vi "UHR-Fleezers Control (fpga) - 11.1.vi"() -> ()   [LabVIEW 2012]
doc: "UHR-Fleezers Instrument Control Code (fpga)"
uses:
  <vilib>/Platform/TimedLoop/XDataNode/timing_clust.ctl
  <vilib>/Platform/TimedLoop/XDataNode/nitl_modes.ctl
  <vilib>/Platform/TimedLoop/XDataNode/wakeup.ctl
  <vilib>/rvi/eio/common/nirviEmuTemplateMethod_errors.vi
  <vilib>/rvi/interface/RandomDataEmulation/nirviRandomDataFPGAFIFO.vi
  <vilib>/rvi/interface/RandomDataEmulation/niFpgaRandomDataHandleErrors.vi
  <vilib>/rvi/Emulation/niFpgaSctlEmulationGetInTimedLoop.vi
  <vilib>/rvi/Emulation/niFpgaSctlEmulationGlobalWrite.vi
  <vilib>/rvi/Emulation/niFpgaSctlEmulationRegisterWithScheduler.vi
  <vilib>/rvi/Emulation/niFpgaSctlEmulationScheduler.vi
  <vilib>/Platform/TimedLoop/XDataNode/XDataNode.xnode
  <vilib>/eio/EIONode/EIONode.xnode
  <vilib>/eio/EIOMethodNode/EIOMethodNode.xnode
  <vilib>/rvi/DataTransferAndStorage/Container/XNode/niFpgaContainer.xnode
  <vilib>/rvi/interface/RandomDataEmulation/nirviRandomDataFpgaReadWriteTemplate.vi
  <vilib>/addons/control/pid/fpga.llb/XNode/niFpgaPID.xnode
  <vilib>/Platform/TimedLoop/XDataNode/XDNodeRunTimeDep.lvlib
panel:
  in  "Tab Control":T1(tab)=enum."Force FB"
  in  "Set 3":bool
  in  "Set 2":bool=TRUE
  in  "Set 1":bool=TRUE
  in  "Trap Pos to FIFO":bool
  in  "N of AI1 Int Acq Sets":i16=2 min=1 max=3 step=1
  out "AI Late Counter":u16
  in  "ai count":u32=400
  out "AI late?":bool
  in  "+ phase":bool
  in  "Phase count adjustment":i16
  out "Relative phase":i16
  in  "AI to FIFO":bool
  out "BD1 Frequency Out 1":u64
  out "BD1 Frequency Out 2":u64
  out "Trap Pos FIFO Timeout":u16
  out "Trap AI FIFO Timeout":u16
  in  "Trap FIFO Set Timeout":i32
  in  "Tab Control 2":T2(tab)
  in  "RD":bool
  in  "FB1 output high":i16=3000
  in  "FB1 output low":i16
  in  "D1":i16
  in  "I1":i16=5
  in  "P1":i16=10
  in  "Swap F1 and F2":bool
  in  "Cont. Scan":bool
  in  "Abort scan":bool
  in  "Cycles per step":u64
  in  "Scan BD":bool
  in  "Number of scans":u16
  in  "Scan steps":u64
  in  "Scan freq.  increment":i64
  out "Scanning":bool
  in  "Start scan":bool
  in  "OSK Bd 1":bool
  in  "Reset Bd 1":bool
  in  "PMODE":bool
  in  "Direct RF Box \nCommunication":bool
  in  "Data BD 2":u8 format="%08b"
  in  "Data BD 1":u8 format="%08b"
  in  "Address":u8 format="%02x"
  in  "Update Data":bool
  in  "FPGA Controls\n RF Box":bool
  in  "Number Interlace Cycles":u8=2 min=1 max=3
  in  "Interlace Off Parameters":u8=1 min=1 max=3
  in  "Interlace ON/OFF":bool
  out "DIO Relative phase":i16
  in  "Phase count adjustment (DIO)":i16
  in  "+ phase (DIO)":bool
  out "DIO Late Counter":u16
  out "DIO Late?":bool
  in  "DIO count 1 (ticks)":u32=400
  in  "DIO count 2 (ticks)":u32=400
  in  "DIO count 3 (ticks)":u32=400
  out "AI2 Y Sum Set 2":i16
  out "AI2 Y Sum Set 1":i16
  in  "FB Setpoint Set 1":i16 min=0 step=1
  in  "FB Reset Set 1":bool
  in  "FB On/Off Set 1":bool
  in  "FB Reset Set 2":bool
  in  "FB On/Off Set 2":bool
  in  "FB Setpoint Set 2":i16 min=0 step=1
  out "Scan I":u64
  in  "Amp switch delay":u16=5
  in  "BD 2 Amplitude 1":u16
  in  "BD 1 Amplitude 1":u16
  in  "BD 2 Frequency 1":u64
  in  "BD 1 Frequency 1":u64
  in  "BD 2 Amplitude 2":u16
  in  "BD 1 Amplitude 2":u16
  in  "BD 2 Frequency 2":u64
  in  "BD 1 Frequency 2":u64
  in  "BD 2 Amplitude 3":u16
  in  "BD 1 Amplitude 3":u16
  in  "BD 2 Frequency 3":u64
  in  "BD 1 Frequency 3":u64
  in  "FB2 output high":fxp<+/-,16,1>=0.999969482421875
  in  "FB2 output low":fxp<+/-,16,1>=-1.0
  in  "P2":fxp<+/-,16,8> format="%.11g"
  in  "I2":fxp<+/-,16,8>=10.0 format="%.11g"
  in  "D2":fxp<+/-,16,8> format="%.11g"
  in  "Negate Diff?":bool
  in  "Diff FB Measurement?":bool
  in  "FB Trig Integrate":u32=1
  out "TTrig?":bool
  in  "TTrig Negate Pos":bool=TRUE
  out "Trap Pos FB Int Signal":fxp<+/-,24,9> format="%.18g"
  out "Trap Pos FB Int-Norm Signal":fxp<+/-,16,1> format="%.16g"
  in  "FPGA TTrig Thresh":i64
  in  "FPGA Trap Trig":bool
  out "Trap Pos FB Action":i64
  in  "Trap Pos. FB Offset Factor":i64
  in  "Trap Pos. FB Mult Factor":i64=2
  in  "Trap Pos. FB Reset":bool
  in  "Trap Pos FB Monitor T1 or T2":bool
  in  "AI1 X Scale":u16
  in  "Trap Pos FB Int Count":u16=100
  in  "Trap Pos FB Negate Action":bool
  out "AI1 X Set 2":fxp<+/-,16,1>
  out "AI1 X Set 1":fxp<+/-,16,1>
  in  "Trap Pos. FB SP":fxp<+/-,16,1>
  in  "Force feedback":bool
  out "TTrig Sig":i64
  out "TTrig Fin Thresh":i64
  in  "1D or 2D Scan?":bool
  in  "Abort scan (MCL)":bool
  in  "MCL Scan Axis":bool
  in  "Cont. Scan (MCL)":bool
  out "Scan I (MCL)":u64
  in  "Number of scans (MCL)":u16
  out "Scanning MCL":bool
  in  "Scan steps (MCL)":u64
  in  "Cycles per step (MCL)":u64
  in  "Scan freq.  increment (MCL)":i16
  in  "Start scan (MCL)":bool
  in  "AO2":i16
  in  "AO1":i16
  out "MCL Late Counter":u16
  out "MCL Late?":bool
  in  "MCL count":u32=800
  out "MCL Relative Phase":i16
  in  "Phase count adjustment (MCL)":i16
  in  "+ phase (MCL)":bool
  in  "APD Gate Operating Mode":u8 max=2 step=1
  in  "Invert APD Gate":bool
  in  "APD Gate OFF Count":u32=100
  in  "APD Gate ON Count":u32=300
  out "APD 1 Gate Late Counter":u16
  out "APD 1 Gate Late?":bool
  out "APD 1 Gate Relative Phase":i16
  in  "Phase count adjustment (APD 1 Gate)":i16
  in  "+ phase (APD 1 Gate)":bool
  out "APD 2 Counts 0":u32
  out "APD 2 Counts 1":u32
  out "APD 1 Counts 0":u32
  out "APD 1 Counts 1":u32
  out "APD1 out state":bool
  in  "APD 2 AO scale factor":i16=1
  in  "APD 1 AO scale factor":i16=1
  in  "APD to FIFO":bool
  in  "APD Acq Rate Count":u32=20000000
  out "APD Acq Late Counter":u16
  out "APD Acq Late?":bool
  out "APD Acq Relative Phase":i16
  in  "Phase Count Adjustment (APD Acq)":i16
  in  "+ phase (APD Acq)":bool
  in  "Phase count adjustment (APD 2 Gate)":i16
  out "APD 2 Gate Late Counter":u16
  out "APD 2 Gate Late?":bool
  out "APD 2 Gate Relative Phase":i16
  in  "+ phase (APD 2 Gate)":bool
  out "APD2 out state":bool
  in  "D3":i16
  in  "I3":i16=5
  in  "P3":i16=10
  in  "Green Filter Flipper":bool
  in  "Green FB Count":u32=1200
  out "Green Late Counter":u16
  out "Green FB Late?":bool
  out "Green FB Relative Phase":i16
  in  "Phase count adjustment (Green FB)":i16=10
  in  "+ phase (Green FB)":bool
  out "Green FB Sum":i16
  in  "Green int current ON count adj":u32=150
  in  "Current Out":u16=30000
  in  "Green FB On/Off":bool
  in  "Green FB Setpoint":i16=250 min=0 step=1
  in  "Green FB Reset":bool
  in  "Operating Mode 2":u8=2 max=2 step=1
  in  "Invert GI 2":bool
  in  "Green interlace OFF count 2":u32=900
  in  "Green interlace ON count 2":u32=300
  out "GI Late Counter 2":u16
  out "GI Late? 2":bool
  out "GI Relative phase 2":i16
  in  "Phase count adjustment (GI) 2":i16=20
  in  "+ phase (GI) 2":bool
  in  "Green interlace OFF count":u32=100
  out "GI Relative phase":i16
  in  "Phase count adjustment (GI)":i16
  in  "+ phase (GI)":bool
  out "GI Late?":bool
  in  "Green interlace ON count":u32=300
  out "GI Late Counter":u16
  in  "Invert GI":bool
  in  "Operating Mode":u8 max=2 step=1
  in  "+ phase (RI)":bool
  out "RI Relative phase":i16
  out "RI Late?":bool
  out "RI Late Counter":u16
  in  "Red interlace ON count":u32=300
  in  "Red interlace OFF count":u32=100
  in  "Invert RI":bool
  in  "Red Laser Operating Mode":u8 max=2 step=1
  in  "Phase count adjustment (RI)":i16
  out "Red FB Intensity":i16
  in  "Phase count adjustment (Red FB)":i16=10
  in  "Red FB Count":u32=1200
  out "Red Late Counter":u16
  out "Red FB Late?":bool
  out "Red FB Relative Phase":i16
  in  "+ phase (Red FB)":bool
  out "Green FB Sum 2":i16
  in  "Phase count adjustment (GI) 3":i16=20
  in  "Green int current ON count adj 2":u32=150
  in  "Current Out 2":u16=30000
  in  "Green FB On/Off 2":bool
  in  "D3 2":i16
  in  "I3 2":i16=5
  in  "P3 2":i16=10
  in  "Green FB Setpoint 2":i16=250 min=0 step=1
  in  "Green FB Reset 2":bool
  in  "Operating Mode 3":u8=2 max=2 step=1
  in  "Invert GI 3":bool
  in  "Green interlace OFF count 3":u32=900
  in  "Green interlace ON count 3":u32=300
  out "GI Late Counter 3":u16
  out "GI Late? 3":bool
  out "GI Relative phase 3":i16
  in  "+ phase (GI) 3":bool
  # "Only one of these can be on\nat a time:"
  # "Raster Scan AOD"
  # "1 (X)"
  # "2 (Y)"
  # "IR Intensity Feedback (RF BD 1)"
  # "FB Gains Set 1"
  # "FB output range 1"
  # "FB Triggering Excitation Laser"
  # "Trap Pos. FB Gains"
  # "Trap Pos. FB Range"
  # "AO1 (Y)"
  # "2D"
  # "1D"
  # "AO2 (X)"
  # "APD AO for aligning"
  # "Detection Loop"
  # "Green fluorescent laser digital gate interlacing loop"
  # "0 Forced ON\n1 Forced OFF\n2 Interlacing"
  # "Green FB Gains"
  # "Red fluorescent laser digital gate interlacing loop"
  # "Detection Loop"
  # "0 Forced ON\n1 Forced OFF\n2 Interlacing"
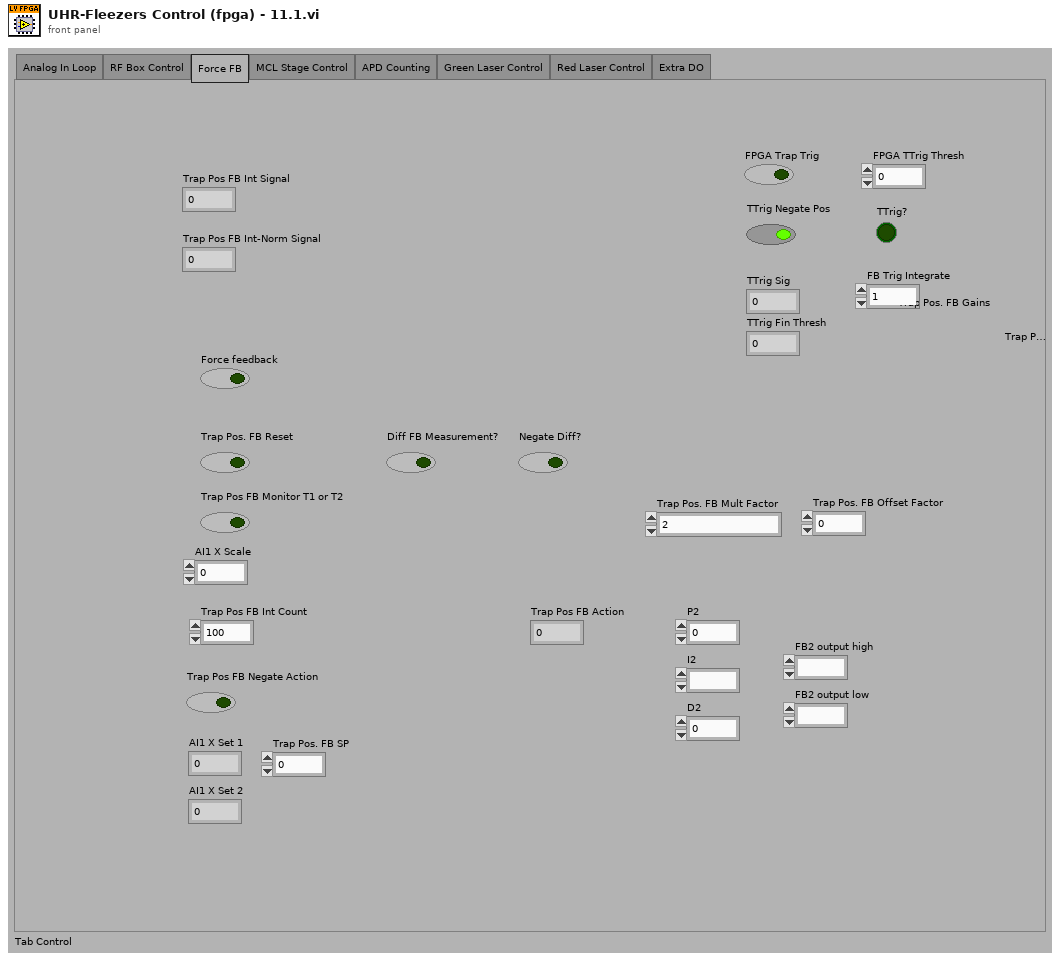
[diagram p1: front panel]
types:
  T1 = enum32{"Analog In Loop", "RF Box Control", "Force FB", "MCL Stage Control", "APD Counting", "Green Laser Control", "Red Laser Control", "Extra DO"}
  T2 = enum32{"Controls", "Interlacing Frequency and Amplitude Values"}
  T3 = typedef "XDNodeRunTimeDep.lvlib/timing_clust.ctl" = cluster{"Expected End [f-1]":u64, "Actual End [f-1]":u64, "Finished Late? [f-1]":bool, "Expected End [i-1]":u64, "Actual End [i-1]":u64, "Finished Late? [i-1]":bool, "Expected Start [i]":u64, "Actual Start [i]":u64, "Expected Start [f]":u64, "Actual Start [f]":u64, "Source Name":string, "Structure Name":string, "Period":i64, "Deadline":i64, "Offset":i64, "Start":i64, "Priority":i32, "Timeout":i32, "Mode":T4, "Wakeup Reason":T5, "Error":errorcluster, "Source Type":string, "Secondary Source Type":string, "Global End Time":u64, "Global Start Time":u64, "Frame Duration":u64, "Iteration Duration":u64, "Assigned CPU":i32, "I/O Scan Engine Mode":u32}
  T4 = typedef "XDNodeRunTimeDep.lvlib/nitl_modes.ctl" = enum32{"No Change", "Process missed periods, maintain original phase", "Discard missed periods, maintain original phase", "Process missed periods, ignore original phase", "Discard missed periods, ignore original phase"}
  T5 = typedef "XDNodeRunTimeDep.lvlib/wakeup.ctl" = enum32{"Normal", "Aborted", "Asynchronous wakeup", "Timing source error", "Timed loop error", "Timeout"}
  T6 = cluster{"proportional gain (Kc)":i16, "integral gain (Kc*Ts/Ti)":i16, "derivative gain (Kc*Td/Ts)":i16}
  T7 = cluster{"FB1 output high":i16, "FB1 output low":i16}
  T8 = cluster{"P2":fxp<+/-,16,8>, "I2":fxp<+/-,16,8>, "D2":fxp<+/-,16,8>}
  T9 = cluster{"FB2 output high":fxp<+/-,16,1>, "FB2 output low":fxp<+/-,16,1>}
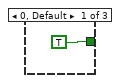
[diagram p3: hidden frame]
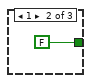
[diagram p4: hidden frame]
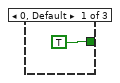
[diagram p5: hidden frame]
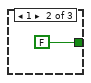
[diagram p6: hidden frame]
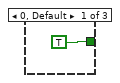
[diagram p7: hidden frame]
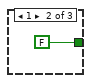
[diagram p8: hidden frame]
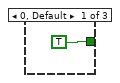
[diagram p10: hidden frame]
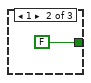
[diagram p11: hidden frame]
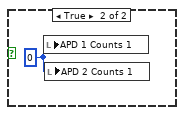
[diagram p12: hidden frame]
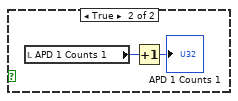
[diagram p14: hidden frame]
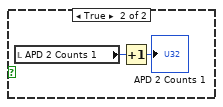
[diagram p15: hidden frame]
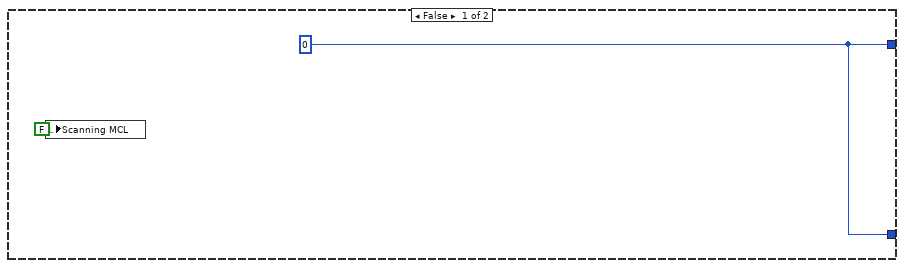
[diagram p16: hidden frame]
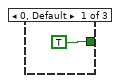
[diagram p17: hidden frame]
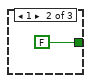
[diagram p18: hidden frame]
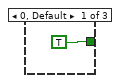
[diagram p19: hidden frame]
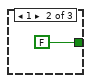
[diagram p20: hidden frame]
diagram:
  w3 = FALSE
  # "timing array current index"
  # "timing array"
  # "timing counter (phase adjusted here)"
  # "late counter"
  n1 = flat-sequence "FPGA initialization to do before running any of the loops" {
    tunnel: [u32 0 ("DIO count 3 (ticks)")] -> w1
    tunnel: [w10] -> _
    frame #0 {
      # "Start up expansion chassis early\nto avoid delays later"
      # "This pin controls udclk on the RF boards.\nWhen initially configuring the boards, this pin needs to be\nconfigured as a high impedance input.  Later it will be switched\nto an output."
      # "Initial setting of DIO data and \naddress to low (before reset).  \nThis needs to happen before the other\ncontrol method loops execute."
      n2 = xnode "FPGA I/O Node"("Chassis2/Mod4/AO0"=u16 0) -> ("Chassis2/Mod1/AI0"=w10:i16)  [unwired: 2 in, 2 out]
      n3 = xnode "FPGA I/O Method Node"("Enable"=FALSE) -> ()  [unwired: 1 in, 1 out]
      n4 = xnode "FPGA I/O Node"("Connector1/DIO0"=FALSE, "Connector1/DIO1"=FALSE, "Connector1/DIO2"=FALSE, "Connector1/DIO3"=FALSE, "Connector1/DIO4"=FALSE, "Connector1/DIO5"=FALSE, "Connector1/DIO6"=FALSE, "Connector1/DIO7"=FALSE, "Connector1/DIO8"=FALSE, "Connector1/DIO9"=FALSE, "Connector1/DIO10"=FALSE, "Connector1/DIO11"=FALSE, "Connector1/DIO12"=FALSE, "Connector1/DIO13"=FALSE, "Connector1/DIO15"=FALSE, "Connector1/DIO20"=FALSE, "Connector1/DIO21"=FALSE, "Connector1/DIO22"=FALSE, "Connector1/DIO23"=FALSE, "Connector1/DIO24"=FALSE, "Connector1/DIO25"=FALSE, "Connector1/DIO26"=FALSE, "Connector1/DIO27"=FALSE, "Connector1/DIO14"=FALSE) -> ()  [unwired: 24 in, 24 out]
    }
  }
  n5 = local read "AO1"() -> (w7:i16)
  n6 = local read "AO2"() -> (w6:i16)
  n7 = node-c288() -> (w5:T3)  [unwired: 1 in]
  n8 = timed-loop "RF box board DIO control: control bits" {
    timing: w5 -> [_]
    timing-out: [_] -> w4
    tunnel: [w40] -> _
    tunnel: w1 -> [w40]
    stop <- FALSE stop-if-true
    n9 = xnode "FPGA I/O Node"("Connector1/DIO16"="RD", "Connector1/DIO17"="PMODE", "Connector1/DIO18"="OSK Bd 1", "Connector1/DIO19"="Reset Bd 1", "Connector0/DIO3"="Green Filter Flipper") -> ()  [unwired: 5 in, 5 out]
  }
  n10 = while "RF box board DIO control: parallel communication" {
    shift-right: [w53] -> _
    shift-left: w1 -> [w52]
    shift-right: [w51] -> _
    shift-left: FALSE ("Swap F1 and F2") -> [w50]
    stop <- FALSE stop-if-true
    n11 = flat-sequence {
      tunnel: w50 -> [w57]
      tunnel: w52 -> [w55]
      tunnel: [w57] -> w49
      tunnel: [w56] -> w48
      tunnel: [w55] -> w47
      tunnel: [w63] -> w53
      tunnel: [w62] -> w51
      tunnel: w49 -> [w61]
      tunnel: w48 -> [w59]
      tunnel: w47 -> [w58]
      frame #0 {
        n12 = call "Loop Timer"("Count(Ticks)"=w55) -> ("Tick Count(Ticks)"=w56:u32)
      }
      frame #1 {
        n13 = flat-sequence {
          tunnel: ["FPGA Controls\n RF Box"] -> w60
          tunnel: w61 -> [w64]
          tunnel: [w104] -> w63
          tunnel: [w117] -> w62
          tunnel: w60 -> [w116]
          tunnel: w59 -> [w110]
          tunnel: w58 -> [w107]
          frame #0 {
            n14 = case shown="True" "FPGA Controls\n RF Box" {
              tunnel: w64 -> [_ w66]
              frame False {
              }
              frame True {
                n15 = flat-sequence {
                  tunnel: w66 -> [w72]
                  frame #0 {
                    n16 = First Call?() -> (First Call?: T/F=w67:bool)
                    n17 = case shown="True" w67 {
                      frame False {
                      }
                      frame True {
                        # "If first time data updated, be sure to set WR high and UDCLK low\nbefore setting data and address bits."
                        n18 = xnode "FPGA I/O Method Node"("Enable"=TRUE) -> ("FPGA I/O Out"=w69:refnum<k21>)  [unwired: 1 in]
                        n19 = xnode "FPGA I/O Node"("Connector1/DIO15"=TRUE) -> ()  [unwired: 1 in, 1 out]
                        n20 = xnode "FPGA I/O Node"("I/O Item"=FALSE ("Connector1/DIO30"), "FPGA I/O In"=w69) -> ()  [unwired: 1 out]
                      }
                    }
                  }
                  frame #1 {
                    n21 = flat-sequence {
                      tunnel: w72 -> [w73]
                      frame #0 {
                        # "switch frequency"
                        n22 = xnode "FPGA I/O Node"("Connector1/DIO36"=w73) -> ()  [unwired: 1 in, 1 out]
                      }
                      frame #1 {
                        n23 = call "Wait4"("Count(Ticks)"="Amp switch delay") -> ()  [unwired: 1 out]
                      }
                      frame #2 {
                        # "switch amplitude"
                        # "send udclk high"
                        n24 = xnode "FPGA I/O Node"("Connector1/DIO30"=TRUE ("Connector1/DIO15")) -> ()  [unwired: 1 in, 1 out]
                      }
                      frame #3 {
                        # "send udclk low"
                        n25 = xnode "FPGA I/O Node"("Connector1/DIO30"=FALSE ("Connector1/DIO15")) -> ()  [unwired: 1 in, 1 out]
                      }
                    }
                  }
                }
              }
            }
          }
          frame #1 {
            # "This is the prior cycle's on time"
            # "increment timing\nindex, reset to 0 if \nend of matrix"
            # "Reset to begginning (1) when number of cycles reached."
            # "timing index"
            # "build byte stacks for writing data\n(must correspond to addresses array constant)"
            # "Timing housekeeping"
            # "Adjust phase if late\n(maintains constant phase relationship between cycles)"
            n26 = Bundle("FB1 output high"="FB1 output high", "FB1 output low"="FB1 output low") -> (w77:T7)  [unwired: 1 in]
            n27 = Bundle("P1"="P1", "I1"="I1", "D1"="D1") -> (w78:cluster{"P1":i16, "I1":i16, "D1":i16})  [unwired: 1 in]
            n28 = feedback #1(u8 0 ("t")) -> (w113:u8)
            n29 = Increment(x=w113) -> (x+1=w157:u8)
            n30 = Increment(x="Number Interlace Cycles") -> (x+1=w152:u8)
            n31 = Equal?(x=w157, y=w152) -> (x = y?=w159:bool)
            n32 = Select(t=u8 1, s=w159, f=w157) -> (s? t:f=w112:u8)
            n33 = feedback-in #1(w112) -> ()
            n34 = Increment(x=w112) -> (x+1=w154:u8)
            n35 = Equal?(x=w154, y=w152) -> (x = y?=w155:bool)
            n36 = Select(t=u8 1, s=w155, f=w154) -> (s? t:f=w151:u8)
            n37 = Select(t=w151, s="Interlace ON/OFF", f="Interlace Off Parameters") -> (s? t:f=w135:u8)
            n38 = case shown="1, Default" w135 {
              tunnel: [w231 "BD 1 Frequency 2" "BD 1 Frequency 3"] -> w147
              tunnel: [w230 "BD 2 Frequency 2" "BD 2 Frequency 3"] -> w136
              tunnel: ["BD 2 Amplitude 1" "BD 2 Amplitude 2" "BD 2 Amplitude 3"] -> w92
              tunnel: [w219 w390 "BD 1 Amplitude 3"] -> w95
              tunnel: w78 -> [w193 w387 _]
              tunnel: w77 -> [w194 w386 _]
              frame 1, Default {
                w210 = fxp<+/-,24,9> 0.0 ("AI1 X Set 2")
                w203 = u16 0
                w226 = u64 0 ("f")
                # "This signal integration happens no matter what\nso that correct setpoints can be chosen before \nturning on the FB."
                # "Trap 1"
                n39 = local read "AI1 X Set 2"() -> (w206:fxp<+/-,16,1>)
                n40 = local read "AI1 X Set 1"() -> (w207:fxp<+/-,16,1>)
                n41 = local read "Scanning"() -> (w232:bool)
                n42 = Or(x=w232, y="Start scan") -> (x .or. y?=w224:bool)
                n43 = case shown="False" "Diff FB Measurement?" {
                  tunnel: w206 -> [w240 w249]
                  tunnel: w207 -> [w239 w250]
                  tunnel: [w237 w241] -> w208
                  frame False {
                    n44 = Select(t=w239, s="Trap Pos FB Monitor T1 or T2", f=w240) -> (s? t:f=w237:fxp<+/-,16,1>)
                  }
                  frame True {
                    n45 = Subtract(x=w250, y=w249) -> (x-y=w242:fxp<+/-,17,2>)
                    n46 = Not(x="Negate Diff?") -> (.not. x?=w248:bool)
                    n47 = Boolean To (0,1)(Boolean="Negate Diff?") -> (0, 1=w246:i16)
                    n48 = Boolean To (0,1)(Boolean=w248) -> (0, 1=w247:i16)
                    n49 = Negate(x=w246) -> (-x=w245:i16)
                    n50 = Add(x=w245, y=w247) -> (x+y=w243:i16)
                    n51 = Multiply(x=w243, y=w242) -> (x*y=w241:fxp<+/-,32,17>)
                  }
                }
                n52 = Not(x="Abort scan") -> (.not. x?=w222:bool)
                n53 = And(x=w222, y=w224) -> (x .and. y?=w221:bool)
                n54 = case "For raster scanning" shown="True" w221 {
                  tunnel: [u64 0 w376] -> w227
                  tunnel: "Start scan" -> [_ w361]
                  frame False {
                    n55 = local write "Scanning"(FALSE ("scanning")) -> ()
                  }
                  frame True {
                    w345 = i64 0
                    w344 = u64 0
                    # "scan incr."
                    # "freq. incr. mult."
                    # "count steps"
                    # "count number of cycles"
                    n56 = feedback #2(w344) -> (w373:u64)
                    n57 = Select(t=w344, s=w361, f=w373) -> (s? t:f=w375:u64)
                    n58 = Increment(x=w375) -> (x+1=w372:u64)
                    n59 = Greater?(x="Cycles per step", y=w372) -> (0:w354:bool)
                    n60 = Select(t=w372, s=w354, f=w344) -> (s? t:f=w371:u64)
                    n61 = feedback-in #2(w371) -> ()
                    n62 = feedback #3(w344) -> (w370:u64)
                    n63 = Select(t=w344, s=w361, f=w370) -> (s? t:f=w365:u64)
                    n64 = Increment(x=w365) -> (x+1=w369:u64)
                    n65 = Add(x="Scan steps", y="Scan steps") -> (x+y=w368:u64)
                    n66 = Select(t=w365, s=w354, f=w369) -> (s? t:f=w349:u64)
                    n67 = Greater?(x=w368, y=w349) -> (0:w348:bool)
                    n68 = Select(t=w349, s=w348, f=w344) -> (s? t:f=w366:u64)
                    n69 = feedback-in #3(w366) -> ()
                    n70 = Equal?(x="Scan steps", y=w349) -> (x = y?=w353:bool)
                    n71 = Greater?(x="Scan steps", y=w365) -> (0:w364:bool)
                    n72 = feedback #4(w345) -> (w367:i64)
                    n73 = Select(t=w345, s=w361, f=w367) -> (s? t:f=w351:i64)
                    n74 = Increment(x=w351) -> (x+1=w363:i64)
                    n75 = Decrement(x=w351) -> (x-1=w362:i64)
                    n76 = Select(t=w363, s=w364, f=w362) -> (s? t:f=w352:i64)
                    n77 = Select(t=w351, s=w353, f=w352) -> (s? t:f=w350:i64)
                    n78 = Select(t=w351, s=w354, f=w350) -> (s? t:f=w346:i64)
                    n79 = Select(t=w346, s=w348, f=w345) -> (s? t:f=w347:i64)
                    n80 = feedback-in #4(w347) -> ()
                    n81 = feedback #5(w344) -> (w360:u64)
                    n82 = Select(t=w344, s=w361, f=w360) -> (s? t:f=w356:u64)
                    n83 = Increment(x=w356) -> (x+1=w357:u64)
                    n84 = Select(t=w356, s=w348, f=w357) -> (s? t:f=w355:u64)
                    n85 = Greater?(x="Number of scans", y=w355) -> (0:w341:bool)
                    n86 = Multiply(x="Scan freq.  increment", y=w351) -> (x*y=w376:i64)
                    n87 = Select(t=TRUE, s="Cont. Scan", f=w341) -> (s? t:f=w340:bool)
                    "Scanning" <- w340
                    n88 = Select(t=w355, s=w340, f=w344) -> (s? t:f=w358:u64)
                    n89 = feedback-in #5(w358) -> ()
                    n90 = Increment(x=w355) -> (x+1=→"Scan I":u64)
                  }
                }
                n91 = feedback #6(w203) -> (w202:u16)
                n92 = Increment(x=w202) -> (x+1=w204:u16)
                n93 = Greater Or Equal?(x=w204, y="Trap Pos FB Int Count") -> (x >= y?=w195:bool)
                n94 = Select(t=w203, s=w195, f=w204) -> (s? t:f=w205:u16)
                n95 = feedback-in #6(w205) -> ()
                n96 = feedback #7(w210) -> (w209:fxp<+/-,24,9>)
                n97 = Add(x=w208, y=w209) -> (x+y=w201:fxp<+/-,24,9>)
                n98 = case "For intensity feedback" shown="True" "FB On/Off Set 1" {
                  tunnel: "BD 1 Amplitude 1" -> [w378 _]
                  tunnel: [w378 w382] -> w219
                  tunnel: w194 -> [_ w379]
                  tunnel: w193 -> [_ w380]
                  frame False {
                  }
                  frame True {
                    n99 = local read "AI2 Y Sum Set 1"() -> (w383:i16)
                    n100 = call "Slower PID.vi"("process variable"=w383, "reset?"="FB Reset Set 1", "setpoint"="FB Setpoint Set 1", "PID gains (x 2^8)"=w380, "output range"=w379) -> ("output"=w384:i16)  [unwired: 10 out]
                    n101 = To Unsigned Word Integer(number=w384) -> (unsigned 16bit integer=w382:u16)
                  }
                }
                n102 = Select(t=w210, s=w195, f=w201) -> (s? t:f=w213:fxp<+/-,24,9>)
                n103 = feedback-in #7(w213) -> ()
                n104 = Divide(x=w201, y="Trap Pos FB Int Count") -> (x/y=w196:fxp<+/-,16,1>)
                n105 = feedback #8(fxp<+/-,24,9> 0.0 ("AI1 X Set 2")) -> (w214:fxp<+/-,24,9>)
                n106 = Select(t=w201, s=w195, f=w214) -> (s? t:f=w215:fxp<+/-,24,9>)
                "Trap Pos FB Int Signal" <- w215
                n107 = feedback-in #8(w215) -> ()
                n108 = feedback #9(fxp<+/-,16,1> 0.0 ("Trap Pos FB Int-Norm Signal")) -> (w198:fxp<+/-,16,1>)
                n109 = Select(t=w196, s=w195, f=w198) -> (s? t:f=w197:fxp<+/-,16,1>)
                "Trap Pos FB Int-Norm Signal" <- w197
                n110 = feedback-in #9(w197) -> ()
                n111 = case "For position feedback" shown="True" "Force feedback" {
                  tunnel: [i64 0 w256] -> w216
                  tunnel: w196 -> [_ w253]
                  tunnel: w195 -> [_ w252]
                  frame False {
                  }
                  frame True {
                    n112 = feedback #10(i64 0) -> (w255:i64)
                    n113 = case shown="True" w252 {
                      tunnel: [w257 w271] -> w256
                      tunnel: w255 -> [w257 _]
                      tunnel: w253 -> [_ w265]
                      frame False {
                      }
                      frame True {
                        w275 = u32 0
                        n114 = Bundle("P2"="P2", "I2"="I2", "D2"="D2") -> (w261:T8)  [unwired: 1 in]
                        n115 = Bundle("FB2 output high"="FB2 output high", "FB2 output low"="FB2 output low") -> (w258:T9)  [unwired: 1 in]
                        n116 = xnode ("PID")("process variable"=w265, "reset?"="Trap Pos. FB Reset", "setpoint"="Trap Pos. FB SP", "PID gains"=w261, "output range"=w258) -> ("output"=w287:fxp<+/-,16,1>)
                        n117 = Negate(x=w287) -> (-x=w286:fxp<+/-,17,2>)
                        n118 = Select(t=w286, s="Trap Pos FB Negate Action", f=w287) -> (s? t:f=w283:fxp<+/-,17,2>)
                        n119 = Scale By Power Of 2(n=u32 15, x=u32 1) -> (x*2^n=w280:u32)
                        n120 = Multiply(x=w283, y=w280) -> (x*y=w279:fxp<+/-,17,17>)
                        n121 = To Quad Integer(1:w279) -> (0:w291:i64)
                        "Trap Pos FB Action" <- w291
                        n122 = Multiply(x=w291, y="Trap Pos. FB Mult Factor") -> (x*y=w289:i64)
                        n123 = Add(x=w289, y="Trap Pos. FB Offset Factor") -> (x+y=w271:i64)
                        n124 = feedback #11() -> (w272:i64)  [unwired: 1 in]
                        n125 = Add(x=w271, y=w272) -> (x+y=w269:i64)
                        n126 = feedback #12(w275) -> (w277:u32)
                        n127 = Increment(x=w277) -> (x+1=w266:u32)
                        n128 = Greater Or Equal?(x=w266, y="FB Trig Integrate") -> (x >= y?=w267:bool)
                        n129 = Select(t=i64 0, s=w267, f=w269) -> (s? t:f=w273:i64)
                        n130 = feedback-in #11(w273) -> ()
                        n131 = Select(t=w275, s=w267, f=w266) -> (s? t:f=w276:u32)
                        n132 = feedback-in #12(w276) -> ()
                        n133 = And(x=w267, y="FPGA Trap Trig") -> (x .and. y?=w274:bool)
                        n134 = case "Trap FB trigger excitation laser ON" shown="True" w274 {
                          tunnel: w269 -> [_ w295]
                          tunnel: w266 -> [_ w293]
                          frame False {
                          }
                          frame True {
                            n135 = Not(x="TTrig Negate Pos") -> (.not. x?=w302:bool)
                            n136 = Boolean To (0,1)(Boolean="TTrig Negate Pos") -> (0, 1=w300:i16)
                            n137 = Boolean To (0,1)(Boolean=w302) -> (0, 1=w301:i16)
                            n138 = Negate(x=w300) -> (-x=w299:i16)
                            n139 = Add(x=w299, y=w301) -> (x+y=w298:i16)
                            n140 = Multiply(x=w298, y=w295) -> (x*y=w297:i64)
                            "TTrig Sig" <- w297
                            n141 = Multiply(x="FPGA TTrig Thresh", y=w293) -> (x*y=w294:i64)
                            "TTrig Fin Thresh" <- w294
                            n142 = Greater Or Equal?(x=w297, y=w294) -> (x >= y?=w296:bool)
                            n143 = case shown="True" w296 {
                              frame False {
                              }
                              frame True {
                                w305 = TRUE ("Green FB On/Off")
                                w307 = u8 2 ("Operating Mode")
                                n144 = local write "Operating Mode 2"(w307) -> ()
                                n145 = local write "Operating Mode"(w307) -> ()
                                n146 = local write "Green FB On/Off"(w305) -> ()
                                n147 = local write "FPGA Trap Trig"(FALSE ("FPGA Trap Trig")) -> ()
                                "TTrig?" <- w305
                              }
                            }
                          }
                        }
                      }
                    }
                    n148 = feedback-in #10(w256) -> ()
                  }
                }
                n149 = Select(t=w226, s="Scan BD", f=w227) -> (s? t:f=w225:u64)
                n150 = Select(t=w227, s="Scan BD", f=w226) -> (s? t:f=w228:u64)
                n151 = Add(x=w225, y="BD 2 Frequency 1") -> (x+y=w230:u64)
                n152 = Compound Arithmetic op=ADD("BD 1 Frequency 1", w216, w228) -> (w231:u64)
                "BD1 Frequency Out 1" <- w231
              }
              frame 2 {
                # "Trap 2"
                n153 = case shown="True" "FB On/Off Set 2" {
                  tunnel: [w394 w397] -> w390
                  tunnel: "BD 1 Amplitude 2" -> [w394 _]
                  tunnel: w387 -> [_ w396]
                  tunnel: w386 -> [_ w395]
                  frame False {
                  }
                  frame True {
                    n154 = local read "AI2 Y Sum Set 2"() -> (w400:i16)
                    n155 = call "Slower PID.vi"("process variable"=w400, "reset?"="FB Reset Set 2", "setpoint"="FB Setpoint Set 2", "PID gains (x 2^8)"=w396, "output range"=w395) -> ("output"=w398:i16)  [unwired: 10 out]
                    n156 = To Unsigned Word Integer(number=w398) -> (unsigned 16bit integer=w397:u16)
                  }
                }
                "BD1 Frequency Out 2" <- "BD 1 Frequency 2"
              }
              frame 3 {
                # "Fluorescence period"
              }
            }
            n157 = feedback-in #13(w110) -> ()
            n158 = feedback #13(w110) -> (w109:u32)
            n159 = Select(t=w112, s="Interlace ON/OFF", f="Interlace Off Parameters") -> (s? t:f=w150:u8)
            n160 = Subtract(x=w110, y=w109) -> (x-y=w108:u32)
            n161 = Subtract "The error"(x=w108, y=w107) -> (x-y=w85:u32)
            n162 = case shown="1, Default" w150 {
              tunnel: ["DIO count 1 (ticks)" "DIO count 2 (ticks)" "DIO count 3 (ticks)"] -> w106
              frame 1, Default {
              }
              frame 2 {
              }
              frame 3 {
              }
            }
            n163 = Number To Boolean Array(number=w85) -> (Boolean array=w86:bool[])
            n164 = Or Array Elements(Boolean array=w86) -> (logical OR=w84:bool)
            "DIO Late?" <- w84
            n165 = Boolean To (0,1)(Boolean=w84) -> (0, 1=w91:i16)
            n166 = To Unsigned Word Integer(number=w91) -> (unsigned 16bit integer=w88:u16)
            n167 = feedback #14(u16 0) -> (w89:u16)
            n168 = Add(x=w88, y=w89) -> (x+y=w87:u16)
            "DIO Late Counter" <- w87
            n169 = feedback-in #14(w87) -> ()
            n170 = Subtract(x=w106, y=w85) -> (x-y=w105:u32)
            n171 = Split Number(x=w147) -> (hi(x)=w146:u32, lo(x)=w145:u32)
            n172 = Split Number(x=w136) -> (hi(x)=w141:u32, lo(x)=w140:u32)
            n173 = Boolean To (0,1)(Boolean="+ phase (DIO)") -> (0, 1=w102:i16)
            n174 = Split Number(x=w146) -> (lo(x)=w144:u16)  [unwired: 1 out]
            n175 = Split Number(x=w145) -> (hi(x)=w143:u16, lo(x)=w142:u16)
            n176 = Split Number(x=w141) -> (lo(x)=w139:u16)  [unwired: 1 out]
            n177 = Split Number(x=w140) -> (hi(x)=w138:u16, lo(x)=w137:u16)
            n178 = Split Number(x=w95) -> (hi(x)=w97:u8, lo(x)=w96:u8)
            n179 = Split Number(x=w92) -> (hi(x)=w94:u8, lo(x)=w93:u8)
            n180 = Split Number(x=w144) -> (hi(x)=w134:u8, lo(x)=w133:u8)
            n181 = Split Number(x=w143) -> (hi(x)=w132:u8, lo(x)=w131:u8)
            n182 = Split Number(x=w139) -> (hi(x)=w127:u8, lo(x)=w126:u8)
            n183 = Split Number(x=w142) -> (hi(x)=w130:u8, lo(x)=w129:u8)
            n184 = Split Number(x=w138) -> (hi(x)=w125:u8, lo(x)=w124:u8)
            n185 = Split Number(x=w137) -> (hi(x)=w123:u8, lo(x)=w122:u8)
            n186 = Multiply(x=w102, y="Phase count adjustment (DIO)") -> (x*y=w98:i16)
            n187 = feedback #15(i16 0) -> (w100:i16)
            n188 = Subtract(x=w100, y=w98) -> (x-y=w99:i16)
            "DIO Relative phase" <- w99
            n189 = feedback-in #15(w99) -> ()
            n190 = Add(x=w105, y=w98) -> (x+y=w104:u32)
            n191 = Build Array "BD 1 A Stack"(w97, w96) -> (w119:u8[])
            n192 = Build Array "BD 2 A Stack"(w94, w93) -> (w118:u8[])
            n193 = Build Array "BD 1 nu Stack"(w134, w133, w132, w131, w130, w129) -> (w128:u8[])
            n194 = Build Array "BD 2 nu Stack"(w127, w126, w125, w124, w123, w122) -> (w121:u8[])
            n195 = case shown="2" w135 {
              tunnel: [w185 w188] -> w117
              tunnel: [u8 10 u8 4] -> w120
              tunnel: "Swap F1 and F2" -> [w186 w188]
              frame 2 {
                # "F2"
                n196 = Not(x=w186) -> (.not. x?=w185:bool)
              }
              frame 1, Default {
                # "low chooses F1"
                # "F1"
              }
            }
            n197 = case "If FPGA is controlling (toggling) RF synth" shown="True" w116 {
              tunnel: w128 -> [_ w164]
              tunnel: w121 -> [_ w163]
              tunnel: w120 -> [_ w162]
              tunnel: w119 -> [_ w161]
              tunnel: w118 -> [_ w160]
              frame False {
              }
              frame True {
                # "Write next amp.\n(wait until beginning of next loop iteration to update)"
                n198 = flat-sequence "Update the next F1 and F2 frequency value (the actual frequency won't change until FSK is switched).\nThen load the next amplitude value into buffer, but don't update it until the next cycle." {
                  tunnel: w164 -> [w167]
                  tunnel: w163 -> [w166]
                  tunnel: w162 -> [w165]
                  tunnel: w161 -> [w178]
                  tunnel: w160 -> [w177]
                  frame #0 {
                    n199 = for {
                      tunnel: w167 -> [w173] mode=indexing
                      tunnel: w166 -> [w172] mode=indexing
                      tunnel: w165 -> [w170]
                      i -> [w171]
                      # "Write next freq."
                      n200 = To Unsigned Byte Integer(number=w171) -> (unsigned 8bit integer=w168:u8)
                      n201 = Add(x=w170, y=w168) -> (x+y=w169:u8)
                      n202 = call "write to RF synth bd.vi"("Address Byte"=w169, "BD 2 Byte"=w172, "BD 1 Byte"=w173) -> ()
                    }
                  }
                  frame #1 {
                    # "send udclk high"
                    n203 = xnode "FPGA I/O Node"("Connector1/DIO30"=TRUE ("Connector1/DIO15")) -> ()  [unwired: 1 in, 1 out]
                  }
                  frame #2 {
                    n204 = xnode "FPGA I/O Node"("Connector1/DIO30"=FALSE ("Connector1/DIO15")) -> ()  [unwired: 1 in, 1 out]
                  }
                  frame #3 {
                    n205 = for {
                      tunnel: w178 -> [w184] mode=indexing
                      tunnel: w177 -> [w183] mode=indexing
                      tunnel: u8 33 -> [w181]
                      i -> [w182]
                      n206 = To Unsigned Byte Integer(number=w182) -> (unsigned 8bit integer=w179:u8)
                      n207 = Add(x=w181, y=w179) -> (x+y=w180:u8)
                      n208 = call "write to RF synth bd.vi"("Address Byte"=w180, "BD 2 Byte"=w183, "BD 1 Byte"=w184) -> ()
                    }
                  }
                }
              }
            }
          }
        }
      }
    }
  }
  n209 = while "RF box board direct communication loop" {
    tunnel: w1 -> [_]
    stop <- FALSE stop-if-true
    n210 = case "Whether to use direct communication method (only use one method at a time)" shown="True" "Direct RF Box \nCommunication" {
      frame False {
      }
      frame True {
        n211 = case shown="True" "Update Data" {
          frame False {
          }
          frame True {
            n212 = flat-sequence {
              frame #0 {
                n213 = First Call?() -> (First Call?: T/F=w409:bool)
                n214 = case shown="True" w409 {
                  frame False {
                  }
                  frame True {
                    # "If first time data updated, be sure to set WR high\nbefore setting data and address bits."
                    n215 = flat-sequence {
                      frame #0 {
                        n216 = xnode "FPGA I/O Node"("Connector1/DIO15"=TRUE) -> ()  [unwired: 1 in, 1 out]
                      }
                      frame #1 {
                        n217 = call "Wait"("Count(Ticks)"=u8 40 ("DO Delay 3 (Ticks)")) -> ()  [unwired: 1 out]
                      }
                    }
                  }
                }
              }
              frame #1 {
                n218 = Number To Boolean Array(number="Address") -> (Boolean array=w458:bool[])
                n219 = Number To Boolean Array(number="Data BD 1") -> (Boolean array=w459:bool[])
                n220 = Number To Boolean Array(number="Data BD 2") -> (Boolean array=w428:bool[])
                n221 = Index Array(array=w459, index=7) -> (element=w443:bool)
                n222 = Index Array(array=w459, index=6) -> (element=w442:bool)
                n223 = Index Array(array=w459, index=5) -> (element=w441:bool)
                n224 = Index Array(array=w459, index=4) -> (element=w440:bool)
                n225 = Index Array(array=w459, index=3) -> (element=w439:bool)
                n226 = Index Array(array=w459, index=2) -> (element=w438:bool)
                n227 = Index Array(array=w459, index=1) -> (element=w437:bool)
                n228 = Index Array(array=w459, index=0) -> (element=w436:bool)
                n229 = Index Array(array=w458, index=5) -> (element=w435:bool)
                n230 = Index Array(array=w458, index=4) -> (element=w434:bool)
                n231 = Index Array(array=w458, index=3) -> (element=w433:bool)
                n232 = Index Array(array=w458, index=2) -> (element=w432:bool)
                n233 = Index Array(array=w458, index=1) -> (element=w431:bool)
                n234 = Index Array(array=w458, index=0) -> (element=w430:bool)
                n235 = Index Array(array=w428, index=7) -> (element=w419:bool)
                n236 = Index Array(array=w428, index=6) -> (element=w418:bool)
                n237 = Index Array(array=w428, index=5) -> (element=w417:bool)
                n238 = Index Array(array=w428, index=4) -> (element=w416:bool)
                n239 = Index Array(array=w428, index=3) -> (element=w415:bool)
                n240 = Index Array(array=w428, index=2) -> (element=w414:bool)
                n241 = Index Array(array=w428, index=1) -> (element=w413:bool)
                n242 = Index Array(array=w428, index=0) -> (element=w412:bool)
                n243 = xnode "FPGA I/O Node"("Connector1/DIO0"=w443, "Connector1/DIO1"=w442, "Connector1/DIO2"=w441, "Connector1/DIO3"=w440, "Connector1/DIO4"=w439, "Connector1/DIO5"=w438, "Connector1/DIO6"=w437, "Connector1/DIO7"=w436, "Connector1/DIO8"=w435, "Connector1/DIO9"=w434, "Connector1/DIO10"=w433, "Connector1/DIO11"=w432, "Connector1/DIO12"=w431, "Connector1/DIO13"=w430, "Connector1/DIO20"=w419, "Connector1/DIO21"=w418, "Connector1/DIO22"=w417, "Connector1/DIO23"=w416, "Connector1/DIO24"=w415, "Connector1/DIO25"=w414, "Connector1/DIO26"=w413, "Connector1/DIO27"=w412) -> ()  [unwired: 22 in, 22 out]
              }
              frame #2 {
                # "wait and then apply write signal"
                n244 = call "Wait2"("Count(Ticks)"=u8 40 ("DO Delay 1 (Ticks)")) -> ()  [unwired: 1 out]
              }
              frame #3 {
                # "sending bit low writes data to board buffer"
                n245 = xnode "FPGA I/O Node"("Connector1/DIO15"=FALSE) -> ()  [unwired: 1 in, 1 out]
              }
              frame #4 {
                # "wait then return write signal"
                n246 = call "Wait3"("Count(Ticks)"=u8 40 ("DO Delay 2 (Ticks)")) -> ()  [unwired: 1 out]
              }
              frame #5 {
                # "sending bit high makes ready to\nwrite more data"
                n247 = xnode "FPGA I/O Node"("Connector1/DIO15"=TRUE) -> ()  [unwired: 1 in, 1 out]
              }
            }
          }
        }
      }
    }
  }
  n248 = while "APD 1 Counter" {
    tunnel: w1 -> [_]
    stop <- FALSE stop-if-true
    n249 = flat-sequence {
      frame #0 {
        n250 = xnode "FPGA I/O Method Node"("FPGA I/O In"=refnum<k21> "Connector0/DIO0" ("APD 1 DO"), "Timeout"=-1) -> ()  [unwired: 2 out]
      }
      frame #1 {
        n251 = local read "APD1 out state"() -> (w469:bool)
        n252 = case shown="False" w469 {
          frame False {
            n253 = local read "APD 1 Counts 0"() -> (w471:u32)
            n254 = Increment(x=w471) -> (x+1=→"APD 1 Counts 0":u32)
          }
          frame True {
            n255 = local read "APD 1 Counts 1"() -> (w473:u32)
            n256 = Increment(x=w473) -> (x+1=→"APD 1 Counts 1":u32)
          }
        }
      }
    }
  }
  n257 = while "APD 2 Counter" {
    tunnel: w1 -> [_]
    stop <- FALSE stop-if-true
    n258 = flat-sequence {
      frame #0 {
        n259 = xnode "FPGA I/O Method Node"("FPGA I/O In"=refnum<k21> "Connector0/DIO1" ("APD 2 DO"), "Timeout"=-1) -> ()  [unwired: 2 out]
      }
      frame #1 {
        n260 = local read "APD2 out state"() -> (w477:bool)
        n261 = case shown="False" w477 {
          frame False {
            n262 = local read "APD 2 Counts 0"() -> (w479:u32)
            n263 = Increment(x=w479) -> (x+1=→"APD 2 Counts 0":u32)
          }
          frame True {
            n264 = local read "APD 2 Counts 1"() -> (w481:u32)
            n265 = Increment(x=w481) -> (x+1=→"APD 2 Counts 1":u32)
          }
        }
      }
    }
  }
  n266 = while "APD 2 Gating" {
    shift-right: [w485] -> _
    shift-left: w1 -> [w490]
    shift-right: [w484] -> _
    shift-left: w3 -> [w482]
    stop <- FALSE stop-if-true
    n267 = flat-sequence {
      tunnel: w490 -> [w493]
      tunnel: [w494] -> w488
      tunnel: [w493] -> w486
      tunnel: [w492] -> w483
      tunnel: w482 -> [w492]
      tunnel: [w497] -> w489
      tunnel: w488 -> [w497]
      tunnel: [w496] -> w487
      tunnel: w486 -> [w496]
      tunnel: w483 -> [w495]
      tunnel: [w515] -> w485
      tunnel: w489 -> [w526]
      tunnel: w487 -> [w524]
      tunnel: [w519] -> w484
      frame #0 {
        n268 = call "Loop Timer8"("Count(Ticks)"=w493) -> ("Tick Count(Ticks)"=w494:u32)
      }
      frame #1 {
        # "(need 4 channels/APD)"
        n269 = xnode "FPGA I/O Node"("Connector0/DIO8"=w495, "Connector0/DIO9"=w495, "Connector0/DIO10"=w495, "Connector0/DIO11"=w495) -> ()  [unwired: 4 in, 4 out]
      }
      frame #2 {
        n270 = local read "APD Gate ON Count"() -> (w508:u32)
        n271 = local read "APD Gate OFF Count"() -> (w507:u32)
        n272 = feedback #16(TRUE) -> (w521:bool)
        n273 = feedback-in #17(w526) -> ()
        n274 = feedback #17(w526) -> (w509:u32)
        n275 = Not(x=w521) -> (.not. x?=w518:bool)
        n276 = feedback-in #16(w518) -> ()
        n277 = Subtract(x=w526, y=w509) -> (x-y=w525:u32)
        n278 = Select(t=w508, s=w518, f=w507) -> (s? t:f=w523:u32)
        n279 = Subtract(x=w525, y=w524) -> (x-y=w500:u32)
        n280 = Subtract(x=w523, y=w500) -> (x-y=w514:u32)
        n281 = Number To Boolean Array(number=w500) -> (Boolean array=w499:bool[])
        n282 = Or Array Elements(Boolean array=w499) -> (logical OR=w498:bool)
        "APD 2 Gate Late?" <- w498
        n283 = Boolean To (0,1)(Boolean="+ phase (APD 2 Gate)") -> (0, 1=w512:i16)
        n284 = Multiply(x=w512, y="Phase count adjustment (APD 2 Gate)") -> (x*y=w510:i16)
        n285 = Boolean To (0,1)(Boolean=w498) -> (0, 1=w505:i16)
        n286 = Add(x=w514, y=w510) -> (x+y=w515:u32)
        n287 = To Unsigned Word Integer(number=w505) -> (unsigned 16bit integer=w502:u16)
        n288 = feedback #18(i16 0) -> (w517:i16)
        n289 = Subtract(x=w517, y=w510) -> (x-y=w516:i16)
        "APD 2 Gate Relative Phase" <- w516
        n290 = feedback-in #18(w516) -> ()
        n291 = feedback #19(u16 0) -> (w503:u16)
        n292 = Add(x=w502, y=w503) -> (x+y=w501:u16)
        "APD 2 Gate Late Counter" <- w501
        n293 = feedback-in #19(w501) -> ()
        n294 = local read "APD Gate Operating Mode"() -> (w506:u8)
        n295 = case shown="2" w506 {
          tunnel: [TRUE FALSE w532] -> w519
          tunnel: w521 -> [_ _ w530]
          frame 0, Default {
          }
          frame 1 {
          }
          frame 2 {
            n296 = local read "Invert APD Gate"() -> (w529:bool)
            n297 = Not(x=w530) -> (.not. x?=w531:bool)
            n298 = Select(t=w531, s=w529, f=w530) -> (s? t:f=w532:bool)
          }
        }
      }
    }
  }
  n299 = while "DAQ AI set 1" {
    shift-right: [w533] -> _
    shift-left: w1 -> [w538]
    stop <- FALSE stop-if-true
    n300 = flat-sequence {
      tunnel: w538 -> [w548]
      tunnel: [w549] -> w536
      tunnel: [w548] -> w535
      tunnel: [w559] -> w546
      tunnel: [w558] -> w545
      tunnel: [w557] -> w544
      tunnel: [w556] -> w543
      tunnel: [w555] -> w542
      tunnel: [w554] -> w541
      tunnel: [w553] -> w540
      tunnel: [w552] -> w539
      tunnel: [w551] -> w537
      tunnel: w536 -> [w551]
      tunnel: w535 -> [w550]
      tunnel: [w550] -> w534
      tunnel: [w588] -> w533
      tunnel: w546 -> [w615]
      tunnel: w545 -> [w580]
      tunnel: w544 -> [w581]
      tunnel: w543 -> [w614]
      tunnel: w542 -> [w604]
      tunnel: w541 -> [w603]
      tunnel: w540 -> [w602]
      tunnel: w539 -> [w601]
      tunnel: w537 -> [w598]
      tunnel: w534 -> [w595]
      frame #0 {
        n301 = call "Loop Timer3"("Count(Ticks)"=w548) -> ("Tick Count(Ticks)"=w549:u32)
      }
      frame #1 {
        n302 = xnode "FPGA I/O Node"("Connector1/DIO31"=TRUE ("Connector1/DIO33")) -> ("Connector0/AI0"=w559:i16, "Connector0/AI1"=w558:i16, "Connector0/AI2"=w557:i16, "Connector0/AI3"=w556:i16, "Connector0/AI4"=w555:i16, "Connector0/AI5"=w554:i16, "Connector0/AI6"=w553:i16, "Connector0/AI7"=w552:i16)  [unwired: 9 in, 9 out]
      }
      frame #2 {
        w584 = FALSE ("AI to FIFO")
        # "Adjust phase after data acquired if button pressed"
        n303 = feedback #20(i16 1) -> (w607:i16)
        n304 = Increment(x=w607) -> (x+1=w613:i16)
        n305 = Scale By Power Of 2(n="AI1 X Scale", x=w580) -> (x*2^n=w578:i16)
        n306 = Greater?(x=w613, y="N of AI1 Int Acq Sets") -> (0:w610:bool)
        n307 = Select(t=i16 1, s=w610, f=w613) -> (s? t:f=w612:i16)
        n308 = feedback-in #20(w612) -> ()
        n309 = Divide(x=w578, y=w581) -> (x/y=w577:fxp<+/-,16,1>)
        n310 = feedback #21(w584) -> (w582:bool)
        n311 = feedback #22(w584) -> (w600:bool)
        n312 = case shown="2" w607 {
          tunnel: w581 -> [w638 w645 _]
          tunnel: ["Set 1" "Set 2" "Set 3"] -> w605
          tunnel: ["AI to FIFO" w647 w652] -> w599
          tunnel: w600 -> [_ w647 w652]
          tunnel: ["Trap Pos to FIFO" w646 w651] -> w583
          tunnel: w582 -> [_ w646 w651]
          tunnel: w577 -> [w637 w644 _]
          tunnel: [w636 w642 FALSE] -> w564
          tunnel: [w635 w643 u64 0 ("BD1 Frequency Out 2")] -> w563
          frame 1, Default {
            n313 = local read "BD1 Frequency Out 1"() -> (w635:u64)
            n314 = Compound Arithmetic op=AND("Trap Pos to FIFO", "Set 1", "AI to FIFO") -> (w636:bool)
            "AI2 Y Sum Set 1" <- w638
            "AI1 X Set 1" <- w637
          }
          frame 2 {
            n315 = local read "BD1 Frequency Out 2"() -> (w643:u64)
            n316 = Compound Arithmetic op=AND(w646, "Set 2", w647) -> (w642:bool)
            "AI2 Y Sum Set 2" <- w645
            "AI1 X Set 2" <- w644
          }
          frame 3 {
          }
        }
        n317 = And(x=w605, y=w599) -> (x .and. y?=w606:bool)
        n318 = case shown="True" w606 {
          tunnel: w615 -> [_ w666]
          tunnel: w580 -> [_ w665]
          tunnel: w581 -> [_ w664]
          tunnel: w614 -> [_ w663]
          tunnel: w604 -> [_ w662]
          tunnel: w603 -> [_ w661]
          tunnel: w602 -> [_ w660]
          tunnel: w601 -> [_ w659]
          tunnel: 0 ("DMA buffer timeout") -> [_ w668]
          frame False {
          }
          frame True {
            n319 = Build Array(w666, w665, w664, w663, w662, w661, w660, w659) -> (w667:i16[])
            n320 = for {
              tunnel: w667 -> [w670] mode=indexing
              tunnel: w668 -> [w671]
              tunnel: [w669] -> w657 mode=indexing
              n321 = xnode ("FIFO Write")("Element"=w670, "Timeout"=w671) -> ("Timed Out?"=w669:bool)  [unwired: 1 in, 1 out]
            }
            n322 = Or Array Elements(Boolean array=w657) -> (logical OR=w654:bool)
            n323 = Boolean To (0,1)(Boolean=w654) -> (0, 1=w656:i16)
            n324 = feedback #23(u16 0) -> (w655:u16)
            n325 = Add(x=w656, y=w655) -> (x+y=w653:u16)
            "Trap AI FIFO Timeout" <- w653
            n326 = feedback-in #23(w653) -> ()
          }
        }
        n327 = feedback-in #21(w583) -> ()
        n328 = feedback-in #22(w599) -> ()
        n329 = case shown="True" w564 {
          tunnel: w563 -> [_ w621]
          tunnel: [u8 0 w618] -> w562
          frame False {
          }
          frame True {
            n330 = Split Number(x=w621) -> (hi(x)=w622:u32, lo(x)=w623:u32)
            n331 = Split Number(x=w622) -> (lo(x)=w624:u16)  [unwired: 1 out]
            n332 = Split Number(x=w623) -> (hi(x)=w625:u16, lo(x)=w626:u16)
            n333 = Build Array "BD 1 nu Stack"(w624, w625, w626) -> (w620:u16[])
            n334 = for {
              tunnel: w620 -> [w633] mode=indexing
              shift-right: [w629] -> w618
              shift-left: u8 0 -> [w630]
              n335 = xnode ("FIFO Method Node")("Element"=w633, "Timeout"="Trap FIFO Set Timeout") -> ("Timed Out?"=w632:bool)  [unwired: 1 in, 1 out]
              n336 = Boolean To (0,1)(Boolean=w632) -> (0, 1=w631:i16)
              n337 = To Unsigned Byte Integer(number=w631) -> (unsigned 8bit integer=w628:u8)
              n338 = Add(x=w628, y=w630) -> (x+y=w629:u8)
            }
          }
        }
        n339 = To Unsigned Word Integer(number=w562) -> (unsigned 16bit integer=w561:u16)
        n340 = feedback #24(u16 0) -> (w575:u16)
        n341 = Add(x=w561, y=w575) -> (x+y=w574:u16)
        "Trap Pos FIFO Timeout" <- w574
        n342 = feedback-in #24(w574) -> ()
        n343 = feedback-in #25(w598) -> ()
        n344 = feedback #25(w598) -> (w597:u32)
        n345 = Subtract(x=w598, y=w597) -> (x-y=w596:u32)
        n346 = xnode "FPGA I/O Node"("Connector1/DIO31"=FALSE ("Connector1/DIO34")) -> ()  [unwired: 1 in, 1 out]
        n347 = Subtract(x=w596, y=w595) -> (x-y=w566:u32)
        n348 = Boolean To (0,1)(Boolean="+ phase") -> (0, 1=w591:i16)
        n349 = Multiply(x=w591, y="Phase count adjustment") -> (x*y=w585:i16)
        n350 = Subtract(x="ai count", y=w566) -> (x-y=w589:u32)
        n351 = Number To Boolean Array(number=w566) -> (Boolean array=w567:bool[])
        n352 = feedback #26(i16 0) -> (w587:i16)
        n353 = Add(x=w589, y=w585) -> (x+y=w588:u32)
        n354 = Subtract(x=w587, y=w585) -> (x-y=w586:i16)
        "Relative phase" <- w586
        n355 = feedback-in #26(w586) -> ()
        n356 = Or Array Elements(Boolean array=w567) -> (logical OR=w565:bool)
        "AI late?" <- w565
        n357 = Boolean To (0,1)(Boolean=w565) -> (0, 1=w572:i16)
        n358 = To Unsigned Word Integer(number=w572) -> (unsigned 16bit integer=w569:u16)
        n359 = feedback #27(u16 0) -> (w570:u16)
        n360 = Add(x=w569, y=w570) -> (x+y=w568:u16)
        "AI Late Counter" <- w568
        n361 = feedback-in #27(w568) -> ()
      }
    }
  }
  n362 = while "MCL stage control" {
    shift-right: [w684] -> _
    shift-left: w1 -> [w687]
    shift-right: [w677] -> _
    shift-left: w7 -> [w674]
    shift-right: [w676] -> _
    shift-left: w6 -> [w672]
    stop <- FALSE stop-if-true
    n363 = flat-sequence {
      tunnel: w687 -> [w691]
      tunnel: [w692] -> w683
      tunnel: [w691] -> w681
      tunnel: [w690] -> w675
      tunnel: w674 -> [w690]
      tunnel: [w689] -> w673
      tunnel: w672 -> [w689]
      tunnel: w683 -> [w696]
      tunnel: [w696] -> w682
      tunnel: w681 -> [w695]
      tunnel: [w695] -> w680
      tunnel: w675 -> [w694]
      tunnel: w673 -> [w693]
      tunnel: w682 -> [w704]
      tunnel: w680 -> [w703]
      tunnel: [w704] -> w686
      tunnel: [w703] -> w685
      tunnel: [w702] -> w679
      tunnel: [w701] -> w678
      tunnel: [w776] -> w684
      tunnel: w686 -> [w783]
      tunnel: w685 -> [w780]
      tunnel: w679 -> [w778]
      tunnel: w678 -> [w777]
      tunnel: [w778] -> w677
      tunnel: [w777] -> w676
      frame #0 {
        n364 = call "Loop Timer5"("Count(Ticks)"=w691) -> ("Tick Count(Ticks)"=w692:u32)
      }
      frame #1 {
        n365 = xnode "FPGA I/O Node"("Connector0/AO1"=w694, "Connector0/AO2"=w693) -> ()  [unwired: 2 in, 2 out]
      }
      frame #2 {
        n366 = local read "Scanning MCL"() -> (w716:bool)
        n367 = Or(x=w716, y="Start scan (MCL)") -> (x .or. y?=w711:bool)
        n368 = Not(x="Abort scan (MCL)") -> (.not. x?=w709:bool)
        n369 = And(x=w709, y=w711) -> (x .and. y?=w708:bool)
        n370 = case "Raster scan" shown="True" w708 {
          tunnel: [w717 w760] -> w713
          tunnel: "Start scan (MCL)" -> [_ w745]
          tunnel: [w717 w721] -> w697
          frame False {
            w717 = i16 0
            n371 = local write "Scanning MCL"(FALSE ("scanning")) -> ()
          }
          frame True {
            w731 = i16 0
            w730 = u64 0
            # "scan incr."
            # "freq. incr. mult."
            # "count steps"
            # "count number of cycles"
            n372 = feedback #28(w730) -> (w757:u64)
            n373 = Select(t=w730, s=w745, f=w757) -> (s? t:f=w759:u64)
            n374 = Increment(x=w759) -> (x+1=w756:u64)
            n375 = Greater?(x="Cycles per step (MCL)", y=w756) -> (0:w740:bool)
            n376 = Select(t=w756, s=w740, f=w730) -> (s? t:f=w755:u64)
            n377 = feedback-in #28(w755) -> ()
            n378 = feedback #29(w730) -> (w754:u64)
            n379 = Select(t=w730, s=w745, f=w754) -> (s? t:f=w749:u64)
            n380 = Increment(x=w749) -> (x+1=w753:u64)
            n381 = Add(x="Scan steps (MCL)", y="Scan steps (MCL)") -> (x+y=w752:u64)
            n382 = Select(t=w749, s=w740, f=w753) -> (s? t:f=w735:u64)
            n383 = Greater?(x=w752, y=w735) -> (0:w734:bool)
            n384 = Select(t=w735, s=w734, f=w730) -> (s? t:f=w750:u64)
            n385 = feedback-in #29(w750) -> ()
            n386 = Equal?(x="Scan steps (MCL)", y=w735) -> (x = y?=w739:bool)
            n387 = Greater?(x="Scan steps (MCL)", y=w749) -> (0:w748:bool)
            n388 = feedback #30(w731) -> (w751:i16)
            n389 = Select(t=w731, s=w745, f=w751) -> (s? t:f=w737:i16)
            n390 = Increment(x=w737) -> (x+1=w747:i16)
            n391 = Decrement(x=w737) -> (x-1=w746:i16)
            n392 = Select(t=w747, s=w748, f=w746) -> (s? t:f=w738:i16)
            n393 = Select(t=w737, s=w739, f=w738) -> (s? t:f=w736:i16)
            n394 = Select(t=w737, s=w740, f=w736) -> (s? t:f=w732:i16)
            n395 = Select(t=w732, s=w734, f=w731) -> (s? t:f=w733:i16)
            n396 = feedback-in #30(w733) -> ()
            n397 = feedback #31(w730) -> (w744:u64)
            n398 = Select(t=w730, s=w745, f=w744) -> (s? t:f=w719:u64)
            n399 = Increment(x=w719) -> (x+1=w741:u64)
            n400 = Select(t=w719, s=w734, f=w741) -> (s? t:f=w720:u64)
            n401 = Greater?(x="Number of scans (MCL)", y=w720) -> (0:w727:bool)
            n402 = Multiply(x="Scan freq.  increment (MCL)", y=w737) -> (x*y=w760:i16)
            n403 = Select(t=TRUE, s="Cont. Scan (MCL)", f=w727) -> (s? t:f=w726:bool)
            "Scanning MCL" <- w726
            n404 = Select(t=w720, s=w726, f=w730) -> (s? t:f=w742:u64)
            n405 = feedback-in #31(w742) -> ()
            n406 = Increment(x=w720) -> (x+1=→"Scan I (MCL)":u64)
            n407 = To Word Integer(number=w719) -> (16bit integer=w722:i16)
            n408 = Multiply(x=w722, y="Scan freq.  increment (MCL)") -> (x*y=w721:i16)
          }
        }
        n409 = Select(t=w697, s="1D or 2D Scan?", f=i16 0) -> (s? t:f=w698:i16)
        n410 = Select(t=w698, s="MCL Scan Axis", f=w713) -> (s? t:f=w712:i16)
        n411 = Select(t=w713, s="MCL Scan Axis", f=w698) -> (s? t:f=w714:i16)
        n412 = Add(x=w712, y="AO2") -> (x+y=w701:i16)
        n413 = Add(x="AO1", y=w714) -> (x+y=w702:i16)
      }
      frame #3 {
        n414 = feedback-in #32(w783) -> ()
        n415 = feedback #32(w783) -> (w782:u32)
        n416 = Boolean To (0,1)(Boolean="+ phase (MCL)") -> (0, 1=w774:i16)
        n417 = Subtract(x=w783, y=w782) -> (x-y=w781:u32)
        n418 = Multiply(x=w774, y="Phase count adjustment (MCL)") -> (x*y=w770:i16)
        n419 = Subtract(x=w781, y=w780) -> (x-y=w762:u32)
        n420 = Subtract(x="MCL count", y=w762) -> (x-y=w772:u32)
        n421 = feedback #33(i16 0) -> (w771:i16)
        n422 = Subtract(x=w771, y=w770) -> (x-y=w769:i16)
        "MCL Relative Phase" <- w769
        n423 = feedback-in #33(w769) -> ()
        n424 = Number To Boolean Array(number=w762) -> (Boolean array=w763:bool[])
        n425 = Or Array Elements(Boolean array=w763) -> (logical OR=w761:bool)
        "MCL Late?" <- w761
        n426 = Boolean To (0,1)(Boolean=w761) -> (0, 1=w768:i16)
        n427 = Add(x=w772, y=w770) -> (x+y=w776:u32)
        n428 = To Unsigned Word Integer(number=w768) -> (unsigned 16bit integer=w765:u16)
        n429 = feedback #34(u16 0) -> (w766:u16)
        n430 = Add(x=w765, y=w766) -> (x+y=w764:u16)
        "MCL Late Counter" <- w764
        n431 = feedback-in #34(w764) -> ()
      }
    }
  }
  n432 = while "APD 1 Gating" {
    shift-right: [w788] -> _
    shift-left: w1 -> [w793]
    shift-right: [w787] -> _
    shift-left: w3 -> [w785]
    stop <- FALSE stop-if-true
    n433 = flat-sequence {
      tunnel: w793 -> [w796]
      tunnel: [w797] -> w791
      tunnel: [w796] -> w789
      tunnel: [w795] -> w786
      tunnel: w785 -> [w795]
      tunnel: [w800] -> w792
      tunnel: w791 -> [w800]
      tunnel: [w799] -> w790
      tunnel: w789 -> [w799]
      tunnel: w786 -> [w798]
      tunnel: [w814] -> w788
      tunnel: w792 -> [w829]
      tunnel: w790 -> [w826]
      tunnel: [w818] -> w787
      frame #0 {
        n434 = call "Loop Timer7"("Count(Ticks)"=w796) -> ("Tick Count(Ticks)"=w797:u32)
      }
      frame #1 {
        # "(need 4 channels/APD)"
        n435 = xnode "FPGA I/O Node"("Connector0/DIO4"=w798, "Connector0/DIO5"=w798, "Connector0/DIO6"=w798, "Connector0/DIO7"=w798) -> ()  [unwired: 4 in, 4 out]
      }
      frame #2 {
        n436 = feedback #35(TRUE) -> (w821:bool)
        n437 = feedback-in #36(w829) -> ()
        n438 = feedback #36(w829) -> (w828:u32)
        n439 = Not(x=w821) -> (.not. x?=w817:bool)
        n440 = feedback-in #35(w817) -> ()
        n441 = Subtract(x=w829, y=w828) -> (x-y=w827:u32)
        n442 = Select(t="APD Gate ON Count", s=w817, f="APD Gate OFF Count") -> (s? t:f=w823:u32)
        n443 = Subtract(x=w827, y=w826) -> (x-y=w802:u32)
        n444 = Subtract(x=w823, y=w802) -> (x-y=w813:u32)
        n445 = Number To Boolean Array(number=w802) -> (Boolean array=w803:bool[])
        n446 = Or Array Elements(Boolean array=w803) -> (logical OR=w801:bool)
        "APD 1 Gate Late?" <- w801
        n447 = Boolean To (0,1)(Boolean="+ phase (APD 1 Gate)") -> (0, 1=w811:i16)
        n448 = Boolean To (0,1)(Boolean=w801) -> (0, 1=w808:i16)
        n449 = Multiply(x=w811, y="Phase count adjustment (APD 1 Gate)") -> (x*y=w809:i16)
        n450 = To Unsigned Word Integer(number=w808) -> (unsigned 16bit integer=w805:u16)
        n451 = Add(x=w813, y=w809) -> (x+y=w814:u32)
        n452 = feedback #37(i16 0) -> (w816:i16)
        n453 = Subtract(x=w816, y=w809) -> (x-y=w815:i16)
        "APD 1 Gate Relative Phase" <- w815
        n454 = feedback-in #37(w815) -> ()
        n455 = feedback #38(u16 0) -> (w806:u16)
        n456 = Add(x=w805, y=w806) -> (x+y=w804:u16)
        "APD 1 Gate Late Counter" <- w804
        n457 = feedback-in #38(w804) -> ()
        n458 = case shown="2" "APD Gate Operating Mode" {
          tunnel: [TRUE FALSE w835] -> w818
          tunnel: w821 -> [_ _ w832]
          frame 0, Default {
          }
          frame 1 {
          }
          frame 2 {
            n459 = Not(x=w832) -> (.not. x?=w834:bool)
            n460 = Select(t=w834, s="Invert APD Gate", f=w832) -> (s? t:f=w835:bool)
          }
        }
      }
    }
  }
  n461 = while "Control APD data integration - stream to host" {
    shift-right: [w838] -> _
    shift-left: w1 -> [w843]
    stop <- FALSE stop-if-true
    n462 = flat-sequence {
      tunnel: w843 -> [w845]
      tunnel: [w846] -> w841
      tunnel: [w845] -> w839
      tunnel: [w854] -> w842
      tunnel: w841 -> [w854]
      tunnel: [w853] -> w840
      tunnel: w839 -> [w853]
      tunnel: [w852] -> w837
      tunnel: [w851] -> w836
      tunnel: [w888] -> w838
      tunnel: w842 -> [w900]
      tunnel: w840 -> [w897]
      tunnel: w837 -> [w881]
      tunnel: w836 -> [w880]
      frame #0 {
        n463 = call "Loop Timer6"("Count(Ticks)"=w845) -> ("Tick Count(Ticks)"=w846:u32)
      }
      frame #1 {
        n464 = flat-sequence {
          tunnel: [w856] -> w850
          tunnel: w850 -> [w858]
          tunnel: [w860] -> w849
          tunnel: [w859] -> w848
          tunnel: [w858] -> w847
          tunnel: [w866] -> w851
          tunnel: [w867] -> w852
          tunnel: w849 -> [w867]
          tunnel: w848 -> [w866]
          tunnel: w847 -> [w865]
          frame #0 {
            # "use two separate variable so each APD won't\nhave to wait to read"
            n465 = feedback #39(FALSE) -> (w855:bool)
            "APD1 out state" <- w855
            "APD2 out state" <- w855
            n466 = Not(x=w855) -> (.not. x?=w856:bool)
            n467 = feedback-in #39(w856) -> ()
          }
          frame #1 {
            n468 = local read "APD 1 Counts 1"() -> (w864:u32)
            n469 = local read "APD 1 Counts 0"() -> (w863:u32)
            n470 = local read "APD 2 Counts 1"() -> (w862:u32)
            n471 = local read "APD 2 Counts 0"() -> (w861:u32)
            n472 = Select(t=w864, s=w858, f=w863) -> (s? t:f=w860:u32)
            n473 = Select(t=w862, s=w858, f=w861) -> (s? t:f=w859:u32)
          }
          frame #2 {
            n474 = case shown="False" w865 {
              frame False {
                w868 = u32 0 ("APD 1 Counts 0")
                n475 = local write "APD 1 Counts 0"(w868) -> ()
                n476 = local write "APD 2 Counts 0"(w868) -> ()
              }
              frame True {
                w869 = u32 0 ("APD 1 Counts 1")
                n477 = local write "APD 1 Counts 1"(w869) -> ()
                n478 = local write "APD 2 Counts 1"(w869) -> ()
              }
            }
          }
        }
      }
      frame #2 {
        n479 = feedback-in #40(w900) -> ()
        n480 = feedback #40(w900) -> (w899:u32)
        n481 = Subtract(x=w900, y=w899) -> (x-y=w898:u32)
        n482 = Subtract(x=w898, y=w897) -> (x-y=w873:u32)
        n483 = case shown="True" "APD to FIFO" {
          tunnel: w881 -> [_ w903]
          tunnel: w880 -> [_ w901]
          frame False {
          }
          frame True {
            n484 = flat-sequence {
              tunnel: 0 ("Timeout") -> [w905]
              tunnel: w903 -> [w906]
              tunnel: [w905] -> w902
              tunnel: w902 -> [w908]
              tunnel: w901 -> [w907]
              frame #0 {
                n485 = xnode ("FIFO Write")("Element"=w906, "Timeout"=w905) -> ()  [unwired: 1 in, 2 out]
              }
              frame #1 {
                n486 = xnode ("FIFO Write")("Element"=w907, "Timeout"=w908) -> ()  [unwired: 1 in, 2 out]
              }
            }
          }
        }
        n487 = Subtract(x="APD Acq Rate Count", y=w873) -> (x-y=w889:u32)
        n488 = Number To Boolean Array(number=w873) -> (Boolean array=w874:bool[])
        n489 = Or Array Elements(Boolean array=w874) -> (logical OR=w872:bool)
        "APD Acq Late?" <- w872
        n490 = Boolean To (0,1)(Boolean=w872) -> (0, 1=w879:i16)
        n491 = To Unsigned Word Integer(number=w879) -> (unsigned 16bit integer=w876:u16)
        n492 = Boolean To (0,1)(Boolean="+ phase (APD Acq)") -> (0, 1=w885:i16)
        n493 = feedback #41(u16 0) -> (w877:u16)
        n494 = Add(x=w876, y=w877) -> (x+y=w875:u16)
        "APD Acq Late Counter" <- w875
        n495 = feedback-in #41(w875) -> ()
        n496 = Multiply(x=w885, y="Phase Count Adjustment (APD Acq)") -> (x*y=w882:i16)
        n497 = Add(x=w889, y=w882) -> (x+y=w888:u32)
        n498 = feedback #42(i16 0) -> (w887:i16)
        n499 = Subtract(x=w887, y=w882) -> (x-y=w884:i16)
        "APD Acq Relative Phase" <- w884
        n500 = feedback-in #42(w884) -> ()
        n501 = To Word Integer(number=w881) -> (16bit integer=w890:i16)
        n502 = To Word Integer(number=w880) -> (16bit integer=w891:i16)
        n503 = Multiply(x="APD 1 AO scale factor", y=w890) -> (x*y=w871:i16)
        n504 = Multiply(x="APD 2 AO scale factor", y=w891) -> (x*y=w870:i16)
        n505 = xnode "FPGA I/O Node"("Connector0/AO5"=w871, "Connector0/AO7"=w870) -> ()  [unwired: 2 in, 2 out]
      }
    }
  }
  n506 = while "532 nm green fluorescent laser interlacing (DO to IA 532 nm AOM ME amp)." {
    shift-right: [w912] -> _
    shift-left: w1 -> [w917]
    shift-right: [w911] -> _
    shift-left: FALSE -> [w909]
    stop <- FALSE stop-if-true
    n507 = flat-sequence {
      tunnel: w917 -> [w920]
      tunnel: [w921] -> w915
      tunnel: [w920] -> w913
      tunnel: [w919] -> w910
      tunnel: w909 -> [w919]
      tunnel: [w924] -> w916
      tunnel: w915 -> [w924]
      tunnel: [w923] -> w914
      tunnel: w913 -> [w923]
      tunnel: w910 -> [w922]
      tunnel: [w933] -> w912
      tunnel: w916 -> [w953]
      tunnel: w914 -> [w950]
      tunnel: [w942] -> w911
      frame #0 {
        n508 = call "Loop Timer4"("Count(Ticks)"=w920) -> ("Tick Count(Ticks)"=w921:u32)
      }
      frame #1 {
        n509 = xnode "FPGA I/O Node"("Connector1/DIO37"=w922, "Connector1/DIO38"=w922, "Connector1/DIO39"=w922) -> ()  [unwired: 3 in, 3 out]
      }
      frame #2 {
        n510 = feedback-in #43(w953) -> ()
        n511 = feedback #43(w953) -> (w952:u32)
        n512 = Subtract(x=w953, y=w952) -> (x-y=w951:u32)
        n513 = Subtract(x=w951, y=w950) -> (x-y=w926:u32)
        n514 = Number To Boolean Array(number=w926) -> (Boolean array=w927:bool[])
        n515 = Or Array Elements(Boolean array=w927) -> (logical OR=w925:bool)
        "GI Late?" <- w925
        n516 = Boolean To (0,1)(Boolean="+ phase (GI)") -> (0, 1=w938:i16)
        n517 = Multiply(x=w938, y="Phase count adjustment (GI)") -> (x*y=w935:i16)
        n518 = Boolean To (0,1)(Boolean=w925) -> (0, 1=w932:i16)
        n519 = To Unsigned Word Integer(number=w932) -> (unsigned 16bit integer=w929:u16)
        n520 = feedback #44(i16 0) -> (w936:i16)
        n521 = feedback #45(u16 0) -> (w930:u16)
        n522 = Add(x=w929, y=w930) -> (x+y=w928:u16)
        "GI Late Counter" <- w928
        n523 = feedback-in #45(w928) -> ()
        n524 = Subtract(x=w936, y=w935) -> (x-y=w934:i16)
        "GI Relative phase" <- w934
        n525 = feedback-in #44(w934) -> ()
        n526 = feedback #46(TRUE) -> (w945:bool)
        n527 = case shown="2" "Operating Mode" {
          tunnel: [TRUE FALSE w959] -> w942
          tunnel: w945 -> [_ _ w956]
          frame 0, Default {
          }
          frame 1 {
          }
          frame 2 {
            n528 = Not(x=w956) -> (.not. x?=w958:bool)
            n529 = Select(t=w958, s="Invert GI", f=w956) -> (s? t:f=w959:bool)
          }
        }
        n530 = Not(x=w945) -> (.not. x?=w941:bool)
        n531 = Select(t="Green interlace ON count", s=w941, f="Green interlace OFF count") -> (s? t:f=w947:u32)
        n532 = Subtract(x=w947, y=w926) -> (x-y=w939:u32)
        n533 = Add(x=w939, y=w935) -> (x+y=w933:u32)
        n534 = feedback-in #46(w941) -> ()
      }
    }
  }
  n535 = while "Green fluorescent laser interlacing (Current to IA 532 nm AOM ME amp)." {
    shift-right: [w965] -> _
    shift-left: w1 -> [w968]
    shift-right: [w962] -> _
    shift-left: u16 0 -> [w960]
    stop <- FALSE stop-if-true
    n536 = flat-sequence {
      tunnel: w968 -> [w971]
      tunnel: [w972] -> w967
      tunnel: [w971] -> w966
      tunnel: [w970] -> w961
      tunnel: w960 -> [w970]
      tunnel: [w975] -> w964
      tunnel: w967 -> [w975]
      tunnel: [w974] -> w963
      tunnel: w966 -> [w974]
      tunnel: w961 -> [w973]
      tunnel: [w984] -> w965
      tunnel: [w1001] -> w962
      tunnel: w964 -> [w1014]
      tunnel: w963 -> [w1011]
      frame #0 {
        n537 = call "Loop Timer10"("Count(Ticks)"=w971) -> ("Tick Count(Ticks)"=w972:u32)
      }
      frame #1 {
        n538 = xnode "FPGA I/O Node"("Chassis2/Mod4/AO0"=w973) -> ()  [unwired: 1 in, 1 out]
      }
      frame #2 {
        n539 = Subtract(x="Green interlace OFF count 2", y="Green int current ON count adj") -> (x-y=w993:u32)
        n540 = feedback-in #47(w1014) -> ()
        n541 = feedback #47(w1014) -> (w1013:u32)
        n542 = Add(x="Green int current ON count adj", y="Green interlace ON count 2") -> (x+y=w994:u32)
        n543 = Subtract(x=w1014, y=w1013) -> (x-y=w1012:u32)
        n544 = Subtract(x=w1012, y=w1011) -> (x-y=w977:u32)
        n545 = Number To Boolean Array(number=w977) -> (Boolean array=w978:bool[])
        n546 = Boolean To (0,1)(Boolean="+ phase (GI) 2") -> (0, 1=w990:i16)
        n547 = Or Array Elements(Boolean array=w978) -> (logical OR=w976:bool)
        "GI Late? 2" <- w976
        n548 = Boolean To (0,1)(Boolean=w976) -> (0, 1=w983:i16)
        n549 = Multiply(x=w990, y="Phase count adjustment (GI) 2") -> (x*y=w986:i16)
        n550 = To Unsigned Word Integer(number=w983) -> (unsigned 16bit integer=w979:u16)
        n551 = feedback #48(u16 0) -> (w981:u16)
        n552 = Add(x=w979, y=w981) -> (x+y=w980:u16)
        "GI Late Counter 2" <- w980
        n553 = feedback-in #48(w980) -> ()
        n554 = feedback #49(i16 0) -> (w987:i16)
        n555 = Subtract(x=w987, y=w986) -> (x-y=w985:i16)
        "GI Relative phase 2" <- w985
        n556 = feedback-in #49(w985) -> ()
        n557 = feedback #50(TRUE) -> (w1006:bool)
        n558 = case shown="2" "Operating Mode 2" {
          tunnel: [TRUE FALSE w1034] -> w995
          tunnel: w1006 -> [_ _ w1031]
          frame 0, Default {
          }
          frame 1 {
          }
          frame 2 {
            n559 = Not(x=w1031) -> (.not. x?=w1033:bool)
            n560 = Select(t=w1033, s="Invert GI 2", f=w1031) -> (s? t:f=w1034:bool)
          }
        }
        n561 = And(x=w995, y="Green FB On/Off") -> (x .and. y?=w996:bool)
        n562 = case shown="True" w996 {
          tunnel: "Current Out" -> [w1015 _]
          tunnel: [w1015 w1024] -> w1000
          frame False {
          }
          frame True {
            n563 = local read "Green FB Sum"() -> (w1020:i16)
            n564 = Bundle("P3"="P3", "I3"="I3", "D3"="D3") -> (w1016:cluster{"P3":i16, "I3":i16, "D3":i16})  [unwired: 1 in]
            n565 = call "Slower PID.vi"("process variable"=w1020, "reset?"="Green FB Reset", "setpoint"="Green FB Setpoint", "PID gains (x 2^8)"=w1016, "output range"=cluster{"output high":i16, "output low":i16} {"output high"=32767, "output low"=-32768} ("Green FB output range")) -> ("output"=w1027:i16)  [unwired: 10 out]
            n566 = To Long Integer(number=w1027) -> (32bit integer=w1021:i32)
            n567 = Add(x=w1021, y=32768) -> (x+y=w1023:i32)
            n568 = To Unsigned Word Integer(number=w1023) -> (unsigned 16bit integer=w1024:u16)
          }
        }
        n569 = Not(x=w1006) -> (.not. x?=w1003:bool)
        n570 = Select(t=w994, s=w1003, f=w993) -> (s? t:f=w1008:u32)
        n571 = Subtract(x=w1008, y=w977) -> (x-y=w988:u32)
        n572 = Add(x=w988, y=w986) -> (x+y=w984:u32)
        n573 = feedback-in #50(w1003) -> ()
        n574 = Boolean To (0,1)(Boolean=w995) -> (0, 1=w1002:i16)
        n575 = To Unsigned Word Integer(number=w1002) -> (unsigned 16bit integer=w999:u16)
        n576 = Multiply(x=w999, y=w1000) -> (x*y=w1001:u16)
      }
    }
  }
  n577 = while "532 nm green excitation laser intensity feedback measurement" {
    shift-right: [w1035] -> _
    shift-left: w1 -> [w1040]
    stop <- FALSE stop-if-true
    n578 = flat-sequence {
      tunnel: w1040 -> [w1042]
      tunnel: [w1043] -> w1038
      tunnel: [w1042] -> w1036
      tunnel: [w1047] -> w1039
      tunnel: w1038 -> [w1047]
      tunnel: [w1046] -> w1037
      tunnel: w1036 -> [w1046]
      tunnel: [w1059] -> w1035
      tunnel: w1039 -> [w1070]
      tunnel: w1037 -> [w1067]
      frame #0 {
        n579 = call "Loop Timer9"("Count(Ticks)"=w1042) -> ("Tick Count(Ticks)"=w1043:u32)
      }
      frame #1 {
        n580 = xnode "FPGA I/O Node"("Connector1/DIO35"=TRUE) -> ("Chassis2/Mod1/AI1"=→"Green FB Sum":i16)  [unwired: 2 in, 2 out]
      }
      frame #2 {
        n581 = feedback-in #51(w1070) -> ()
        n582 = feedback #51(w1070) -> (w1069:u32)
        n583 = Subtract(x=w1070, y=w1069) -> (x-y=w1068:u32)
        n584 = xnode "FPGA I/O Node"("Connector1/DIO35"=FALSE) -> ()  [unwired: 1 in, 1 out]
        n585 = Subtract(x=w1068, y=w1067) -> (x-y=w1049:u32)
        n586 = Subtract(x="Green FB Count", y=w1049) -> (x-y=w1063:u32)
        n587 = Number To Boolean Array(number=w1049) -> (Boolean array=w1050:bool[])
        n588 = Or Array Elements(Boolean array=w1050) -> (logical OR=w1048:bool)
        "Green FB Late?" <- w1048
        n589 = Boolean To (0,1)(Boolean="+ phase (Green FB)") -> (0, 1=w1061:i16)
        n590 = Boolean To (0,1)(Boolean=w1048) -> (0, 1=w1055:i16)
        n591 = Multiply(x=w1061, y="Phase count adjustment (Green FB)") -> (x*y=w1056:i16)
        n592 = Add(x=w1063, y=w1056) -> (x+y=w1059:u32)
        n593 = To Unsigned Word Integer(number=w1055) -> (unsigned 16bit integer=w1052:u16)
        n594 = feedback #52(i16 0) -> (w1058:i16)
        n595 = Subtract(x=w1058, y=w1056) -> (x-y=w1057:i16)
        "Green FB Relative Phase" <- w1057
        n596 = feedback-in #52(w1057) -> ()
        n597 = feedback #53(u16 0) -> (w1053:u16)
        n598 = Add(x=w1052, y=w1053) -> (x+y=w1051:u16)
        "Green Late Counter" <- w1051
        n599 = feedback-in #53(w1051) -> ()
      }
    }
  }
  n600 = node-c288(w4) -> ()
  n601 = while "Red fluorescent laser interlacing (Current to IA 532 nm AOM ME amp)." {
    shift-right: [w1076] -> _
    shift-left: _ -> [w1079]
    shift-right: [w1073] -> _
    shift-left: _ -> [w1071]
    stop <- FALSE stop-if-true
    n602 = flat-sequence {
      tunnel: w1079 -> [w1082]
      tunnel: [w1083] -> w1078
      tunnel: [w1082] -> w1077
      tunnel: [w1081] -> w1072
      tunnel: w1071 -> [w1081]
      tunnel: [w1086] -> w1075
      tunnel: w1078 -> [w1086]
      tunnel: [w1085] -> w1074
      tunnel: w1077 -> [w1085]
      tunnel: w1072 -> [w1084]
      tunnel: [w1095] -> w1076
      tunnel: [w1112] -> w1073
      tunnel: w1075 -> [w1125]
      tunnel: w1074 -> [w1122]
      frame #0 {
        n603 = call "Loop Timer2"("Count(Ticks)"=w1082) -> ("Tick Count(Ticks)"=w1083:u32)
      }
      frame #1 {
        n604 = xnode "FPGA I/O Node"("Chassis2/Mod4/AO0"=w1084) -> ()  [unwired: 1 in, 1 out]
      }
      frame #2 {
        n605 = Subtract(x="Green interlace OFF count 3", y="Green int current ON count adj 2") -> (x-y=w1104:u32)
        n606 = feedback-in #54(w1125) -> ()
        n607 = feedback #54(w1125) -> (w1124:u32)
        n608 = Add(x="Green int current ON count adj 2", y="Green interlace ON count 3") -> (x+y=w1105:u32)
        n609 = Subtract(x=w1125, y=w1124) -> (x-y=w1123:u32)
        n610 = Subtract(x=w1123, y=w1122) -> (x-y=w1088:u32)
        n611 = Number To Boolean Array(number=w1088) -> (Boolean array=w1089:bool[])
        n612 = Boolean To (0,1)(Boolean="+ phase (GI) 3") -> (0, 1=w1101:i16)
        n613 = Or Array Elements(Boolean array=w1089) -> (logical OR=w1087:bool)
        "GI Late? 3" <- w1087
        n614 = Boolean To (0,1)(Boolean=w1087) -> (0, 1=w1094:i16)
        n615 = Multiply(x=w1101, y="Phase count adjustment (GI) 3") -> (x*y=w1097:i16)
        n616 = To Unsigned Word Integer(number=w1094) -> (unsigned 16bit integer=w1090:u16)
        n617 = feedback #55(u16 0) -> (w1092:u16)
        n618 = Add(x=w1090, y=w1092) -> (x+y=w1091:u16)
        "GI Late Counter 3" <- w1091
        n619 = feedback-in #55(w1091) -> ()
        n620 = feedback #56(i16 0) -> (w1098:i16)
        n621 = Subtract(x=w1098, y=w1097) -> (x-y=w1096:i16)
        "GI Relative phase 3" <- w1096
        n622 = feedback-in #56(w1096) -> ()
        n623 = feedback #57(TRUE) -> (w1117:bool)
        n624 = case shown="2" "Operating Mode 3" {
          tunnel: [TRUE FALSE w1145] -> w1106
          tunnel: w1117 -> [_ _ w1142]
          frame 0, Default {
          }
          frame 1 {
          }
          frame 2 {
            n625 = Not(x=w1142) -> (.not. x?=w1144:bool)
            n626 = Select(t=w1144, s="Invert GI 3", f=w1142) -> (s? t:f=w1145:bool)
          }
        }
        n627 = And(x=w1106, y="Green FB On/Off 2") -> (x .and. y?=w1107:bool)
        n628 = case shown="True" w1107 {
          tunnel: "Current Out 2" -> [w1126 _]
          tunnel: [w1126 w1135] -> w1111
          frame False {
          }
          frame True {
            n629 = local read "Green FB Sum 2"() -> (w1131:i16)
            n630 = Bundle("P3 2"="P3 2", "I3 2"="I3 2", "D3 2"="D3 2") -> (w1127:cluster{"P3 2":i16, "I3 2":i16, "D3 2":i16})  [unwired: 1 in]
            n631 = call "Slower PID.vi"("process variable"=w1131, "reset?"="Green FB Reset 2", "setpoint"="Green FB Setpoint 2", "PID gains (x 2^8)"=w1127, "output range"=cluster{"output high":i16, "output low":i16} {"output high"=32767, "output low"=-32768} ("Green FB output range")) -> ("output"=w1138:i16)  [unwired: 10 out]
            n632 = To Long Integer(number=w1138) -> (32bit integer=w1132:i32)
            n633 = Add(x=w1132, y=32768) -> (x+y=w1134:i32)
            n634 = To Unsigned Word Integer(number=w1134) -> (unsigned 16bit integer=w1135:u16)
          }
        }
        n635 = Not(x=w1117) -> (.not. x?=w1114:bool)
        n636 = Select(t=w1105, s=w1114, f=w1104) -> (s? t:f=w1119:u32)
        n637 = Subtract(x=w1119, y=w1088) -> (x-y=w1099:u32)
        n638 = Add(x=w1099, y=w1097) -> (x+y=w1095:u32)
        n639 = feedback-in #57(w1114) -> ()
        n640 = Boolean To (0,1)(Boolean=w1106) -> (0, 1=w1113:i16)
        n641 = To Unsigned Word Integer(number=w1113) -> (unsigned 16bit integer=w1110:u16)
        n642 = Multiply(x=w1110, y=w1111) -> (x*y=w1112:u16)
      }
    }
  }
  n643 = while "633 nm red excitation laser intensity feedback measurement" {
    shift-right: [w1146] -> _
    shift-left: w1 -> [w1151]
    stop <- FALSE stop-if-true
    n644 = flat-sequence {
      tunnel: w1151 -> [w1153]
      tunnel: [w1154] -> w1149
      tunnel: [w1153] -> w1147
      tunnel: [w1158] -> w1150
      tunnel: w1149 -> [w1158]
      tunnel: [w1157] -> w1148
      tunnel: w1147 -> [w1157]
      tunnel: [w1170] -> w1146
      tunnel: w1150 -> [w1181]
      tunnel: w1148 -> [w1178]
      frame #0 {
        n645 = call "Loop Timer12"("Count(Ticks)"=w1153) -> ("Tick Count(Ticks)"=w1154:u32)
      }
      frame #1 {
        n646 = xnode "FPGA I/O Node"("Connector1/DIO29"=TRUE ("Connector1/DIO35")) -> ("Chassis2/Mod1/AI2"=→"Red FB Intensity":i16)  [unwired: 2 in, 2 out]
      }
      frame #2 {
        n647 = feedback-in #58(w1181) -> ()
        n648 = feedback #58(w1181) -> (w1180:u32)
        n649 = Subtract(x=w1181, y=w1180) -> (x-y=w1179:u32)
        n650 = xnode "FPGA I/O Node"("Connector1/DIO29"=FALSE ("Connector1/DIO35")) -> ()  [unwired: 1 in, 1 out]
        n651 = Subtract(x=w1179, y=w1178) -> (x-y=w1160:u32)
        n652 = Subtract(x="Red FB Count", y=w1160) -> (x-y=w1174:u32)
        n653 = Number To Boolean Array(number=w1160) -> (Boolean array=w1161:bool[])
        n654 = Or Array Elements(Boolean array=w1161) -> (logical OR=w1159:bool)
        "Red FB Late?" <- w1159
        n655 = Boolean To (0,1)(Boolean="+ phase (Red FB)") -> (0, 1=w1172:i16)
        n656 = Boolean To (0,1)(Boolean=w1159) -> (0, 1=w1166:i16)
        n657 = Multiply(x=w1172, y="Phase count adjustment (Red FB)") -> (x*y=w1167:i16)
        n658 = Add(x=w1174, y=w1167) -> (x+y=w1170:u32)
        n659 = To Unsigned Word Integer(number=w1166) -> (unsigned 16bit integer=w1163:u16)
        n660 = feedback #59(i16 0) -> (w1169:i16)
        n661 = Subtract(x=w1169, y=w1167) -> (x-y=w1168:i16)
        "Red FB Relative Phase" <- w1168
        n662 = feedback-in #59(w1168) -> ()
        n663 = feedback #60(u16 0) -> (w1164:u16)
        n664 = Add(x=w1163, y=w1164) -> (x+y=w1162:u16)
        "Red Late Counter" <- w1162
        n665 = feedback-in #60(w1162) -> ()
      }
    }
  }
  n666 = while "633 nm red  fluorescent laser interlacing (DO to IA 633 nm AOM ME amp)." {
    shift-right: [w1185] -> _
    shift-left: w1 -> [w1190]
    shift-right: [w1184] -> _
    shift-left: _ -> [w1182]
    stop <- FALSE stop-if-true
    n667 = flat-sequence {
      tunnel: w1190 -> [w1193]
      tunnel: [w1194] -> w1188
      tunnel: [w1193] -> w1186
      tunnel: [w1192] -> w1183
      tunnel: w1182 -> [w1192]
      tunnel: [w1197] -> w1189
      tunnel: w1188 -> [w1197]
      tunnel: [w1196] -> w1187
      tunnel: w1186 -> [w1196]
      tunnel: w1183 -> [w1195]
      tunnel: [w1206] -> w1185
      tunnel: w1189 -> [w1226]
      tunnel: w1187 -> [w1223]
      tunnel: [w1215] -> w1184
      frame #0 {
        n668 = call "Loop Timer11"("Count(Ticks)"=w1193) -> ("Tick Count(Ticks)"=w1194:u32)
      }
      frame #1 {
        n669 = xnode "FPGA I/O Node"("Connector1/DIO32"=w1195, "Connector1/DIO33"=w1195, "Connector1/DIO34"=w1195) -> ()  [unwired: 3 in, 3 out]
      }
      frame #2 {
        n670 = feedback-in #61(w1226) -> ()
        n671 = feedback #61(w1226) -> (w1225:u32)
        n672 = Subtract(x=w1226, y=w1225) -> (x-y=w1224:u32)
        n673 = Subtract(x=w1224, y=w1223) -> (x-y=w1199:u32)
        n674 = Number To Boolean Array(number=w1199) -> (Boolean array=w1200:bool[])
        n675 = Or Array Elements(Boolean array=w1200) -> (logical OR=w1198:bool)
        "RI Late?" <- w1198
        n676 = Boolean To (0,1)(Boolean="+ phase (RI)") -> (0, 1=w1211:i16)
        n677 = Multiply(x=w1211, y="Phase count adjustment (RI)") -> (x*y=w1208:i16)
        n678 = Boolean To (0,1)(Boolean=w1198) -> (0, 1=w1205:i16)
        n679 = To Unsigned Word Integer(number=w1205) -> (unsigned 16bit integer=w1202:u16)
        n680 = feedback #62(i16 0) -> (w1209:i16)
        n681 = feedback #63(u16 0) -> (w1203:u16)
        n682 = Add(x=w1202, y=w1203) -> (x+y=w1201:u16)
        "RI Late Counter" <- w1201
        n683 = feedback-in #63(w1201) -> ()
        n684 = Subtract(x=w1209, y=w1208) -> (x-y=w1207:i16)
        "RI Relative phase" <- w1207
        n685 = feedback-in #62(w1207) -> ()
        n686 = feedback #64(TRUE) -> (w1218:bool)
        n687 = case shown="2" "Red Laser Operating Mode" {
          tunnel: [TRUE FALSE w1232] -> w1215
          tunnel: w1218 -> [_ _ w1229]
          frame 0, Default {
          }
          frame 1 {
          }
          frame 2 {
            n688 = Not(x=w1229) -> (.not. x?=w1231:bool)
            n689 = Select(t=w1231, s="Invert RI", f=w1229) -> (s? t:f=w1232:bool)
          }
        }
        n690 = Not(x=w1218) -> (.not. x?=w1214:bool)
        n691 = Select(t="Red interlace ON count", s=w1214, f="Red interlace OFF count") -> (s? t:f=w1220:u32)
        n692 = Subtract(x=w1220, y=w1199) -> (x-y=w1212:u32)
        n693 = Add(x=w1212, y=w1208) -> (x+y=w1206:u32)
        n694 = feedback-in #64(w1214) -> ()
      }
    }
  }
